vi "Motors.vi"(5 "Motors Active":refnum<vi>, 6 "Cluster":T1, 7 "Set":refnum<vi>, 8 "Error":refnum<vi>, 9 "Scan in Progress":refnum<vi>, 10 "EMERGENCY":refnum<vi>, 11 "QUIT":refnum<vi>) -> ()   [LabVIEW 2018]
uses:
  <vilib>/Utility/error.llb/DialogType.ctl
panel:
  out "Theta (deg)":refnum<vi>
  out "Z (mm)":refnum<vi>
  out "Y (mm)":refnum<vi>
  out "X (mm)":refnum<vi>
  out "Set?":bool
  out "Theta Go?":bool
  out "Z Go?":bool
  out "Y Go?":bool
  out "X Go?":bool
  out "Theta Go To (mm)":refnum<vi>
  out "Z Go To (mm)":refnum<vi>
  out "Y Go To (mm)":refnum<vi>
  out "X Go To (mm)":refnum<vi>
  out "Theta Go":refnum<vi>
  out "Z Go":refnum<vi>
  out "Y Go":refnum<vi>
  out "X Go":refnum<vi>
  out "Loop i":i32
  in  "Motors":enum32{"Controls", "Advanced Settings"}(tab)
  in  "Theta Speed (deg/s)":dbl=1.0 min=0.0
  in  "Z Speed (mm/s)":dbl=1.0 min=0.0
  in  "Y Speed (mm/s)":dbl=1.0 min=0.0
  in  "X Speed (mm/s)":dbl=1.0 min=0.0
  out "Status Z":string
  out "Status Theta":string
  out "Status Y":string
  out "Status X":string
  out "Z-Axis (mm)":dbl
  out "Theta (deg)":dbl
  out "Y-Axis (mm)":dbl
  out "X-Axis (mm)":dbl
  in  "theta+":bool
  in  "theta-":bool
  in  "Theta Go To":dbl
  in  "Theta Go":bool
  in  "x+":bool
  in  "x-":bool
  in  "X Go To":dbl
  in  "X Go":bool
  in  "y+":bool
  in  "y-":bool
  in  "Y Go To":dbl
  in  "Y Go":bool
  in  "z+":bool
  in  "z-":bool
  in  "Z Go To":dbl
  in  "Z Go":bool
  in  "Defined Positions":i32(listbox)
  in  "Go To Saved Position":bool
  in  "Delta X (mm)":dbl=1.0
  in  "Jog-Mode":bool
  in  "Delta Y (mm)":dbl=1.0
  in  "Delta Z (mm)":dbl=1.0
  in  "Delta Theta (deg)":dbl=1.0
  in  "Save New Position":bool
  in  "New Position Name":string
  in  "Delete Position":bool
  in  "Stop X":bool
  in  "Stop Y":bool
  in  "Stop Z":bool
  in  "Stop Theta":bool
  in  "Enable Motors":bool
  out "Motors Online":bool
  out "Motors Status":string
  out "Update Params":bool caption="Updating Motor Parameters"
  out "X Moving":bool caption="X"
  out "Y Moving":bool caption="Y"
  out "Z Moving":bool caption="Z"
  out "Theta Moving":bool caption="Theta"
  in  "Saved Positions":path=path "C:/LabView VIs/IPES SubVIs/saved_positions.txt"
  in  "Saved Limits":path=path "C:/LabView VIs/IPES SubVIs/saved_limits.txt"
  out "Theta Multiplier":u32=100 caption="steps/deg"
  out "Z Multiplier":u32=200 caption="steps/mm"
  out "Y Multiplier":u32=2000 caption="steps/mm"
  out "X Multiplier":u32=2000 caption="steps/mm"
  in  "Set Multipliers":bool
  in  "User Theta Mult":u32=100 caption="Theta" min=1
  in  "User Z Mult":u32=200 caption="Z" min=1
  in  "User Y Mult":u32=2000 caption="Y" min=1
  in  "User X Mult":u32=2000 caption="X" min=1
  in  "Set Joger":bool
  in  "Fast":dbl=200.0
  in  "Jogger Axis":u16(ring) items=["X (mm/s)", "Y (mm/s)", "Z (mm/s)", "Theta (deg/s)"]
  in  "Normal":dbl=200.0
  out "Y Jogger Fast Speed":dbl caption="mm/s"
  out "Y Jogger Normal Speed":dbl caption="mm/s"
  in  "Manual IO":bool
  in  "Reset Motors":bool caption="Load Previously Saved Parameters"
  in  "Redefine Origin":bool caption="Redefine Origin as Current Location"
  in  "Save Params":bool caption="Save Current Motor Parameters"
  in  "Find Datums":bool caption="Find Datums Nearest Hard Limits"
  in  "Use Datums":bool caption="Use Datums Nearest Hard Limits to Reset Origin"
  out "Manual Com":bool caption="Manual Communication is Active\n(Close Window Before Ending Program)"
  out "X Jogger Normal Speed":dbl caption="mm/s"
  out "X Jogger Fast Speed":dbl caption="mm/s"
  out "Z Jogger Normal Speed":dbl caption="mm/s"
  out "Z Jogger Fast Speed":dbl caption="mm/s"
  out "Theta Jogger Normal Speed":dbl caption="deg/s"
  out "Theta Jogger Fast Speed":dbl caption="deg/s"
  in  "Motors Port":refnum<visa-resource-name>="COM10"
  in  "User X Slew Speed":dbl=3.0 caption="X" min=0.4
  in  "User Y Slew Speed":dbl=3.0 caption="Y" min=0.4
  in  "User Z Slew Speed":dbl=2.0 caption="Z" min=0.5
  in  "User Theta Slew Speed":dbl=7.0 caption="Theta" min=1.0
  in  "X Set Slew Speed":bool
  in  "Y Set Slew Speed":bool
  in  "Z Set Slew Speed":bool
  in  "Theta Set Slew Speed":bool
  out "X Slew Speed":dbl caption="mm/s" min=0.0
  out "Y Slew Speed":dbl caption="mm/s" min=0.0
  out "Z Slew Speed":dbl caption="mm/s" min=0.0
  out "Theta Slew Speed":dbl caption="deg/s" min=0.0
  in  "Backlash X":u32=200 caption="X"
  in  "Backlash Y":u32=200 caption="Y"
  in  "Backlash Z":u32=50 caption="Z"
  in  "Backlash Theta":u32=50 caption="Theta"
  in  "Set Backlash":bool
  in  "Steps to Deactivate Hard Limit After Finding Datums":dbl=2000.0
  out "Theta Action":string
  out "Z Action":string
  out "Y Action":string
  out "X Action":string
  # "Status"
  # "Move Distance \n(Step Mode)"
  # "Remote Jogger Speeds"
  # "Encoder Multipliers"
  # "Motor Backlash Steps"
  # "Motor Speeds"
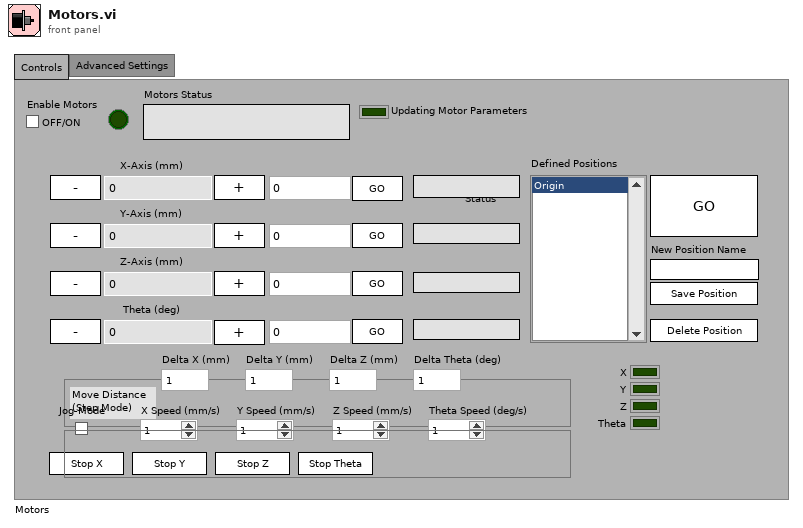
[diagram p1: front panel]
types:
  T1 = cluster{"X Go":refnum<vi>, "Y Go":refnum<vi>, "Z Go":refnum<vi>, "Theta Go":refnum<vi>, "X Go To (mm)":refnum<vi>, "Y Go To (mm)":refnum<vi>, "Z Go To (mm)":refnum<vi>, "Theta Go To (deg)":refnum<vi>, "X (mm)":refnum<vi>, "Y (mm)":refnum<vi>, "Z (mm)":refnum<vi>, "Theta (deg)":refnum<vi>}
  T2 = typedef "DialogType.ctl" = u16
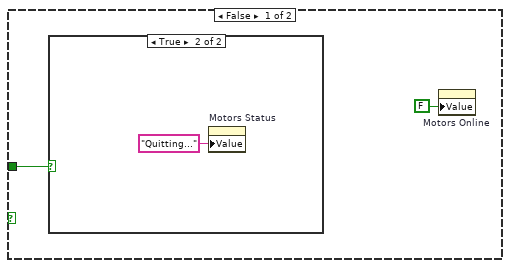
[diagram p2: hidden frame]
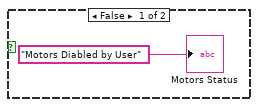
[diagram p3: hidden frame]
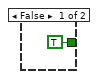
[diagram p10: hidden frame]
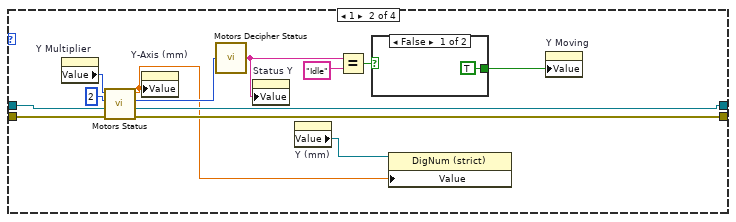
[diagram p11: hidden frame]
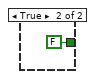
[diagram p12: hidden frame]
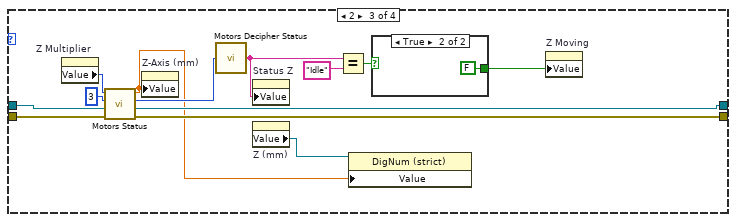
[diagram p13: hidden frame]
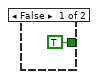
[diagram p14: hidden frame]
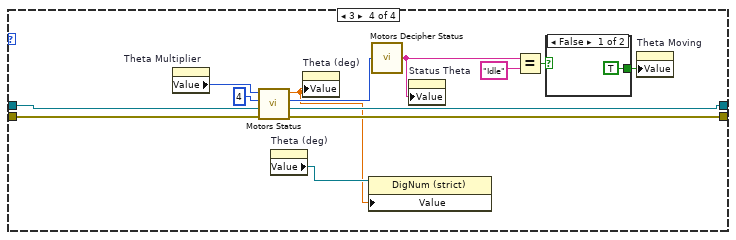
[diagram p15: hidden frame]
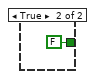
[diagram p16: hidden frame]
diagram:
  n1 = flat-sequence {
    frame #0 {
      w1 = FALSE ("Update Params")
      w2 = FALSE ("Visible")
      n2 = call "Motors Position Load.vi"() -> ("Positions"=w28:string[][])  [unwired: 2 in, 1 out]
      n3 = property on="Scan in Progress" class="LVObjRef (strict)"("Visible"=w2) -> ()  [unwired: 2 in, 2 out]
      n4 = property on="EMERGENCY" class="LVObjRef (strict)"("Visible"=w2) -> ()  [unwired: 2 in, 2 out]
      n5 = property on="Set" class="LVObjRef (strict)"("Visible"=w2) -> ()  [unwired: 2 in, 2 out]
      n6 = property on="Error" class="LVObjRef (strict)"("Visible"=w2) -> ()  [unwired: 2 in, 2 out]
      n7 = property on="Motors Active" class="LVObjRef (strict)"("Visible"=w2) -> ()  [unwired: 2 in, 2 out]
      n8 = property on="QUIT" class="LVObjRef (strict)"("Visible"=w2) -> ()  [unwired: 2 in, 2 out]
      n9 = property on="Loop i" class="DigNum (strict)"("Visible"=w2) -> ()  [unwired: 2 in, 2 out]
      n10 = property on="Set?" class="Bool (strict)"("Visible"=w2) -> ()  [unwired: 2 in, 2 out]
      n11 = property on="Z Go To (mm)" class="LVObjRef (strict)"("Visible"=w2) -> ()  [unwired: 2 in, 2 out]
      n12 = property on="Theta Go To (mm)" class="LVObjRef (strict)"("Visible"=w2) -> ()  [unwired: 2 in, 2 out]
      n13 = property on="Y Go To (mm)" class="LVObjRef (strict)"("Visible"=w2) -> ()  [unwired: 2 in, 2 out]
      n14 = property on="X Go To (mm)" class="LVObjRef (strict)"("Visible"=w2) -> ()  [unwired: 2 in, 2 out]
      n15 = property on="Y Go" class="LVObjRef (strict)"("Visible"=w2) -> ()  [unwired: 2 in, 2 out]
      n16 = property on="X Go" class="LVObjRef (strict)"("Visible"=w2) -> ()  [unwired: 2 in, 2 out]
      n17 = property on="Z Go" class="LVObjRef (strict)"("Visible"=w2) -> ()  [unwired: 2 in, 2 out]
      n18 = property on="Theta Go" class="LVObjRef (strict)"("Visible"=w2) -> ()  [unwired: 2 in, 2 out]
      n19 = property on="Cluster" class="Clust (strict)"("Visible"=w2) -> ()  [unwired: 2 in, 2 out]
      n20 = Array Subset(array=w28, index (row)=0 ("index"), length (row)=1 ("length"), index (col)=0 ("index")) -> (w24:string[][])  [unwired: 1 in]
      n21 = Unbundle("Cluster") -> ("X Go"=→"X Go":refnum<vi>, "Y Go"=→"Y Go":refnum<vi>, "Z Go"=→"Z Go":refnum<vi>, "Theta Go"=→"Theta Go":refnum<vi>, "X Go To (mm)"=→"X Go To (mm)":refnum<vi>, "Y Go To (mm)"=→"Y Go To (mm)":refnum<vi>, "Z Go To (mm)"=→"Z Go To (mm)":refnum<vi>, "Theta Go To (deg)"=→"Theta Go To (mm)":refnum<vi>, "X (mm)"=→"X (mm)":refnum<vi>, "Y (mm)"=→"Y (mm)":refnum<vi>, "Z (mm)"=→"Z (mm)":refnum<vi>, "Theta (deg)"=→"Theta (deg)":refnum<vi>)
      n22 = Initialize Array("", 1 ("dimension size")) -> (w21:string[])
      n23 = Index Array(array=w24) -> (element=w20:string[])  [unwired: 2 in]
      n24 = property on="X (mm)" class="LVObjRef (strict)"("Visible"=w2) -> ()  [unwired: 2 in, 2 out]
      n25 = property on="Z (mm)" class="LVObjRef (strict)"("Visible"=w2) -> ()  [unwired: 2 in, 2 out]
      n26 = property on="Y (mm)" class="LVObjRef (strict)"("Visible"=w2) -> ()  [unwired: 2 in, 2 out]
      n27 = property on="Theta (deg)" class="LVObjRef (strict)"("Visible"=w2) -> ()  [unwired: 2 in, 2 out]
      n28 = Insert Into Array(array=w21, new element=w20) -> (w19:string[])  [unwired: 1 in]
      n29 = property on="Enable Motors" class="Bool (strict)"("Value"=w1) -> ()  [unwired: 2 in, 2 out]
      n30 = property on="Update Params" class="Bool (strict)"("Value"=w1) -> ()  [unwired: 2 in, 2 out]
      n31 = property on="X Go?" class="Bool (strict)"("Visible"=w2) -> ()  [unwired: 2 in, 2 out]
      n32 = property on="Z Go?" class="Bool (strict)"("Visible"=w2) -> ()  [unwired: 2 in, 2 out]
      n33 = property on="Theta Go?" class="Bool (strict)"("Visible"=w2) -> ()  [unwired: 2 in, 2 out]
      n34 = property on="Y Go?" class="Bool (strict)"("Visible"=w2) -> ()  [unwired: 2 in, 2 out]
      n35 = Delete From Array(array=w19, index=0) -> (array with subset deleted=w17:string[])  [unwired: 1 in, 1 out]
      n36 = property on="Defined Positions" class="LstBox (strict)"("Item Names"=w17) -> ()  [unwired: 2 in, 2 out]
      n37 = property on="X Moving" class="Bool (strict)"("Value"=w1) -> ()  [unwired: 2 in, 2 out]
      n38 = property on="Y Moving" class="Bool (strict)"("Value"=w1) -> ()  [unwired: 2 in, 2 out]
      n39 = property on="Theta Moving" class="Bool (strict)"("Value"=w1) -> ()  [unwired: 2 in, 2 out]
      n40 = property on="Z Moving" class="Bool (strict)"("Value"=w1) -> ()  [unwired: 2 in, 2 out]
      "Motors Online" <- FALSE ("Motors Online")
      "Set?" <- FALSE ("Set?")
    }
    frame #1 {
      n41 = while {
        stop <- w36 stop-if-true
        n42 = property on="QUIT" class="LVObjRef (strict)"() -> ("Value"=w32:refnum<vi>)  [unwired: 2 in, 2 out]
        n43 = property class="Bool (strict)"(reference=w32) -> ("Value"=w34:bool)  [unwired: 1 in, 2 out]
        n44 = property class="Bool (strict)"(reference="QUIT") -> ("Value"=w36:bool)  [unwired: 1 in, 2 out]
        n45 = Not(x=w34) -> (.not. x?=w33:bool)
        n46 = And(x=w33, y="Enable Motors") -> (x .and. y?=w31:bool)
        n47 = case shown="True" w31 {
          tunnel: "Enable Motors" -> [w38 _]
          frame False {
            n48 = case shown="True" w38 {
              frame False {
                "Motors Status" <- "Motors Diabled by User" ("Motors Status")
              }
              frame True {
                n49 = property on="Motors Status" class="Str"("Value"="Quitting..." ("Motors Status")) -> ()  [unwired: 2 in, 2 out]
              }
            }
            n50 = property on="Motors Online" class="Bool (strict)"("Value"=FALSE ("Motors Online")) -> ()  [unwired: 2 in, 2 out]
          }
          frame True {
            n51 = call "Motors Open.vi"("VISA in"="Motors Port") -> ("error out"=w43:errorcluster, "VISA out"=w42:refnum<visa-resource-name>)  [unwired: 1 in]
            n52 = case shown="Error" w43 {
              selector: w43 -> [_ w1402]
              tunnel: w42 -> [w51 _]
              frame No Error {
                n53 = while {
                  tunnel: w51 -> [w57]
                  tunnel: [w55] -> w47
                  i -> [w56]
                  stop <- w65 stop-if-true
                  n54 = property on="Enable Motors" class="Bool (strict)"() -> ("Value"=w67:bool)  [unwired: 2 in, 2 out]
                  n55 = property on="QUIT" class="LVObjRef (strict)"() -> ("Value"=w64:refnum<vi>)  [unwired: 2 in, 2 out]
                  n56 = Not(x=w67) -> (.not. x?=w66:bool)
                  n57 = property class="Bool (strict)"(reference=w64) -> ("Value"=w63:bool)  [unwired: 1 in, 2 out]
                  n58 = property class="Bool (strict)"(reference="Scan in Progress") -> ("Value"=w61:bool)  [unwired: 1 in, 2 out]
                  n59 = property class="Bool (strict)"(reference="Set") -> ("Value"=w54:bool)  [unwired: 1 in, 2 out]
                  n60 = Or(x=w66, y=w63) -> (x .or. y?=w65:bool)
                  n61 = Not(x=w61) -> (.not. x?=w59:bool)
                  n62 = Or(x=w59, y=w54) -> (x .or. y?=w58:bool)
                  n63 = case shown="True" w58 {
                    tunnel: w57 -> [w68 w91]
                    tunnel: w56 -> [_ w182]
                    tunnel: [w68 w72] -> w55
                    tunnel: w54 -> [_ w93]
                    frame False {
                    }
                    frame True {
                      # "This loop checks every button consecutively (no particular order) to see if it has been pushed, and then executes the respective motor operation(s).  If a scan is running, the buttons are ignored and no operations are executed.  If the scan has called a <Set> operation, then the indicated motors are set to their indicated positions."
                      n64 = case shown="False" w93 {
                        tunnel: [w430 w436] -> w92
                        tunnel: w91 -> [w430 w436]
                        frame False {
                          # "A scan is not running.  If the user pushes a <# Go> button, then the # motor will move to the user-input position."
                          n65 = case shown="True" "Theta Go" {
                            selector: "Theta Go" -> [_ w432]
                            frame False {
                            }
                            frame True {
                              n66 = property on="Theta Go?" class="Bool (strict)"("Value"=w432) -> ()  [unwired: 2 in, 2 out]
                            }
                          }
                          n67 = case shown="True" "X Go" {
                            selector: "X Go" -> [_ w434]
                            frame False {
                            }
                            frame True {
                              n68 = property on="X Go?" class="Bool (strict)"("Value"=w434) -> ()  [unwired: 2 in, 2 out]
                            }
                          }
                          n69 = case shown="True" "Z Go" {
                            selector: "Z Go" -> [_ w431]
                            frame False {
                            }
                            frame True {
                              n70 = property on="Z Go?" class="Bool (strict)"("Value"=w431) -> ()  [unwired: 2 in, 2 out]
                            }
                          }
                          n71 = case shown="True" "Y Go" {
                            selector: "Y Go" -> [_ w433]
                            frame False {
                            }
                            frame True {
                              n72 = property on="Y Go?" class="Bool (strict)"("Value"=w433) -> ()  [unwired: 2 in, 2 out]
                            }
                          }
                        }
                        frame True {
                          # "<Set?> is a local variable that indicates that the global variable <Set> was True when the motor loop started.  We use it instead of just reading <Set> so as to avoid errors that may happen if another VI changes the state of <Set> part way through the motor loop being executed.  <Set?> will be set to True only if <Set> is True and <Set?> is False, thus the motor loop will execute exactly once."
                          n73 = property on="Set?" class="Bool (strict)"() -> ("Value"=w435:bool)  [unwired: 2 in, 2 out]
                          n74 = case shown="False" w435 {
                            frame False {
                              # "The global variables <# Go> are boolean flags that indacte if the position of the # motor should be set during a <Set> operation.  The global variables <# Go To> indicate the value of said position.  Both are copied to local variables to avoid errors if the the global variables are changed during the motor loop."
                              n75 = property on="Theta Go" class="LVObjRef (strict)"() -> ("Value"=w453:refnum<vi>)  [unwired: 2 in, 2 out]
                              n76 = property on="X Go" class="LVObjRef (strict)"() -> ("Value"=w447:refnum<vi>)  [unwired: 2 in, 2 out]
                              n77 = property on="Z Go" class="LVObjRef (strict)"() -> ("Value"=w451:refnum<vi>)  [unwired: 2 in, 2 out]
                              n78 = property on="Y Go" class="LVObjRef (strict)"() -> ("Value"=w445:refnum<vi>)  [unwired: 2 in, 2 out]
                              n79 = property on="Set?" class="Bool (strict)"("Value"=TRUE ("Set?")) -> ()  [unwired: 2 in, 2 out]
                              n80 = property class="Bool (strict)"(reference=w447) -> ("Value"=→"X Go?":bool)  [unwired: 1 in, 2 out]
                              n81 = property class="Bool (strict)"(reference=w451) -> ("Value"=→"Z Go?":bool)  [unwired: 1 in, 2 out]
                              n82 = property class="Bool (strict)"(reference=w445) -> ("Value"=→"Y Go?":bool)  [unwired: 1 in, 2 out]
                              n83 = property class="Bool (strict)"(reference=w453) -> ("Value"=→"Theta Go?":bool)  [unwired: 1 in, 2 out]
                              n84 = property on="Theta Go To (mm)" class="LVObjRef (strict)"() -> ("Value"=w448:refnum<vi>)  [unwired: 2 in, 2 out]
                              n85 = property on="Z Go To (mm)" class="LVObjRef (strict)"() -> ("Value"=w441:refnum<vi>)  [unwired: 2 in, 2 out]
                              n86 = property on="Y Go To (mm)" class="LVObjRef (strict)"() -> ("Value"=w440:refnum<vi>)  [unwired: 2 in, 2 out]
                              n87 = property on="X Go To (mm)" class="LVObjRef (strict)"() -> ("Value"=w438:refnum<vi>)  [unwired: 2 in, 2 out]
                              n88 = property class="DigNum (strict)"(reference=w441) -> ("Value"=w443:dbl)  [unwired: 1 in, 2 out]
                              n89 = property class="DigNum (strict)"(reference=w448) -> ("Value"=w449:dbl)  [unwired: 1 in, 2 out]
                              n90 = property class="DigNum (strict)"(reference=w440) -> ("Value"=w442:dbl)  [unwired: 1 in, 2 out]
                              n91 = property class="DigNum (strict)"(reference=w438) -> ("Value"=w439:dbl)  [unwired: 1 in, 2 out]
                              n92 = property on="Z Go To" class="DigNum (strict)"("Value"=w443) -> ()  [unwired: 2 in, 2 out]
                              n93 = property on="Theta Go To" class="DigNum (strict)"("Value"=w449) -> ()  [unwired: 2 in, 2 out]
                              n94 = property on="Y Go To" class="DigNum (strict)"("Value"=w442) -> ()  [unwired: 2 in, 2 out]
                              n95 = property on="X Go To" class="DigNum (strict)"("Value"=w439) -> ()  [unwired: 2 in, 2 out]
                            }
                            frame True {
                            }
                          }
                        }
                      }
                      n96 = property on="Error" class="LVObjRef (strict)"() -> ("Value"=w174:refnum<vi>)  [unwired: 2 in, 2 out]
                      n97 = property class="Clust (strict)"(reference=w174) -> ("Value"=w84:errorcluster)  [unwired: 1 in, 2 out]
                      n98 = property on="X Moving" class="Bool (strict)"() -> ("Value"=w98:bool)  [unwired: 2 in, 2 out]
                      n99 = property on="Y Moving" class="Bool (strict)"() -> ("Value"=w97:bool)  [unwired: 2 in, 2 out]
                      n100 = property on="Z Moving" class="Bool (strict)"() -> ("Value"=w96:bool)  [unwired: 2 in, 2 out]
                      n101 = property on="Theta Moving" class="Bool (strict)"() -> ("Value"=w95:bool)  [unwired: 2 in, 2 out]
                      n102 = Compound Arithmetic op=OR(w98, w97, w96, w95) -> (w94:bool)
                      n103 = case shown="False" "Save New Position" {
                        tunnel: w84 -> [w478 w497]
                        tunnel: [w478 w496] -> w103
                        frame False {
                        }
                        frame True {
                          # "Write the current position to file and make visible in the list of positions."
                          n104 = property on="Theta (deg)" class="DigNum (strict)"() -> ("Value"=w480:dbl)  [unwired: 2 in, 2 out]
                          n105 = property on="Saved Positions" class="Path"() -> ("Value"=w499:path)  [unwired: 2 in, 2 out]
                          n106 = property on="X-Axis (mm)" class="DigNum (strict)"() -> ("Value"=w483:dbl)  [unwired: 2 in, 2 out]
                          n107 = property on="Y-Axis (mm)" class="DigNum (strict)"() -> ("Value"=w482:dbl)  [unwired: 2 in, 2 out]
                          n108 = property on="Z-Axis (mm)" class="DigNum (strict)"() -> ("Value"=w481:dbl)  [unwired: 2 in, 2 out]
                          n109 = call "Motors Position Save.vi"("file path"=w499, "error in"=w497, "Position Name"="New Position Name", "Theta (deg)"=w480, "Z (mm)"=w481, "Y (mm)"=w482, "X (mm)"=w483) -> ("error out"=w498:errorcluster)  [unwired: 3 in]
                          n110 = call "Motors Position Load.vi"("error in"=w498, "file path"=w499) -> ("error out"=w496:errorcluster, "Positions"=w484:string[][])
                          n111 = Array Subset(array=w484, index (row)=0 ("index"), length (row)=1 ("length"), index (col)=0 ("index")) -> (w489:string[][])  [unwired: 1 in]
                          n112 = Initialize Array("", 1 ("dimension size")) -> (w490:string[])
                          n113 = Index Array(array=w489) -> (element=w492:string[])  [unwired: 2 in]
                          n114 = Insert Into Array(array=w490, new element=w492) -> (w493:string[])  [unwired: 1 in]
                          n115 = Delete From Array(array=w493, index=0) -> (array with subset deleted=w479:string[])  [unwired: 1 in, 1 out]
                          n116 = property on="Defined Positions" class="LstBox (strict)"("Item Names"=w479) -> ()  [unwired: 2 in, 2 out]
                        }
                      }
                      n117 = property class="Bool (strict)"(reference="Motors Active", "Value"=w94) -> ()  [unwired: 1 in, 2 out]
                      n118 = case shown="False" "Set Multipliers" {
                        frame False {
                        }
                        frame True {
                          # "Multipliers are the ratio of steps to mm (or deg) for each motor.  These are stored as local variables and used only by the GUI, i.e. not by the motor controllers."
                          "X Multiplier" <- "User X Mult"
                          "Y Multiplier" <- "User Y Mult"
                          "Z Multiplier" <- "User Z Mult"
                          "Theta Multiplier" <- "User Theta Mult"
                        }
                      }
                      n119 = case shown="False" "Delete Position" {
                        tunnel: w103 -> [w458 w476]
                        tunnel: [w458 w475] -> w102
                        frame False {
                        }
                        frame True {
                          # "Remove the selected position from the file and the list."
                          n120 = property on="Saved Positions" class="Path"() -> ("Value"=w461:path)  [unwired: 2 in, 2 out]
                          n121 = property on="Defined Positions" class="LstBox (strict)"() -> ("Value"=w460:i32)  [unwired: 2 in, 2 out]
                          n122 = call "Motors Position Load.vi"("error in"=w476, "file path"=w461) -> ("error out"=w477:errorcluster, "Positions"=w474:string[][])
                          n123 = Delete From Array(array=w474, index (col)=w460) -> (array with subset deleted=w473:string[][])  [unwired: 2 in, 1 out]
                          n124 = call "Motors Position Load.vi"("error in"=w477, "file path"=w461) -> ("error out"=w475:errorcluster, "Positions"=w462:string[][])
                          n125 = call "Motors Position Rewrite.vi"("file path"=w461, "Array of Positions"=w473) -> ()  [unwired: 9 in]
                          n126 = Array Subset(array=w462, index (row)=0 ("index"), length (row)=1 ("length"), index (col)=0 ("index")) -> (w467:string[][])  [unwired: 1 in]
                          n127 = Initialize Array("", 1 ("dimension size")) -> (w468:string[])
                          n128 = Index Array(array=w467) -> (element=w470:string[])  [unwired: 2 in]
                          n129 = Insert Into Array(array=w468, new element=w470) -> (w471:string[])  [unwired: 1 in]
                          n130 = Delete From Array(array=w471, index=0) -> (array with subset deleted=w459:string[])  [unwired: 1 in, 1 out]
                          n131 = property on="Defined Positions" class="LstBox (strict)"("Item Names"=w459) -> ()  [unwired: 2 in, 2 out]
                        }
                      }
                      n132 = case shown="False" "Stop X" {
                        tunnel: w102 -> [w1388 w1394]
                        tunnel: w92 -> [w1389 w1393]
                        tunnel: [w1389 w1391] -> w176
                        tunnel: [w1388 w1390] -> w177
                        frame False {
                        }
                        frame True {
                          # "The X motor stops moving immediately."
                          n133 = call "Motors Stop.vi"("error in"=w1394, "Axis"=1, "VISA in"=w1393) -> ("error out"=w1390:errorcluster, "VISA out"=w1391:refnum<visa-resource-name>)
                        }
                      }
                      n134 = case shown="False" "Stop Y" {
                        tunnel: w177 -> [w1381 w1387]
                        tunnel: w176 -> [w1382 w1386]
                        tunnel: [w1382 w1384] -> w178
                        tunnel: [w1381 w1383] -> w179
                        frame False {
                        }
                        frame True {
                          n135 = call "Motors Stop.vi"("error in"=w1387, "Axis"=2, "VISA in"=w1386) -> ("error out"=w1383:errorcluster, "VISA out"=w1384:refnum<visa-resource-name>)
                        }
                      }
                      n136 = case shown="False" "Stop Z" {
                        tunnel: w179 -> [w1374 w1380]
                        tunnel: w178 -> [w1375 w1379]
                        tunnel: [w1375 w1377] -> w180
                        tunnel: [w1374 w1376] -> w181
                        frame False {
                        }
                        frame True {
                          n137 = call "Motors Stop.vi"("error in"=w1380, "Axis"=3, "VISA in"=w1379) -> ("error out"=w1376:errorcluster, "VISA out"=w1377:refnum<visa-resource-name>)
                        }
                      }
                      n138 = case shown="True" "Stop Theta" {
                        tunnel: w181 -> [w1367 w1373]
                        tunnel: w180 -> [w1368 w1372]
                        tunnel: [w1368 w1370] -> w170
                        tunnel: [w1367 w1369] -> w169
                        frame False {
                        }
                        frame True {
                          n139 = call "Motors Stop.vi"("error in"=w1373, "Axis"=4, "VISA in"=w1372) -> ("error out"=w1369:errorcluster, "VISA out"=w1370:refnum<visa-resource-name>)
                        }
                      }
                      n140 = case shown="False" "Set Backlash" {
                        tunnel: [w1358 w1366] -> w166
                        tunnel: w170 -> [w1358 w1365]
                        tunnel: w169 -> [w1357 w1364]
                        tunnel: [w1357 w1363] -> w167
                        frame False {
                        }
                        frame True {
                          # "Set the number of steps to use for backlash correction."
                          n141 = call "Motors Backlash.vi"("X"="Backlash X", "Y"="Backlash Y", "VISA in"=w1365, "error in"=w1364, "Z"="Backlash Z", "Theta"="Backlash Theta") -> ("VISA out"=w1366:refnum<visa-resource-name>, "error out"=w1363:errorcluster)  [unwired: 2 in]
                        }
                      }
                      n142 = Or(x="x+", y="x-") -> (x .or. y?=w138:bool)
                      n143 = case shown="True" "Manual IO" {
                        tunnel: [w1340 w1347] -> w161
                        tunnel: [w1341 w1342] -> w162
                        tunnel: w166 -> [w1341 w1344]
                        tunnel: w167 -> [w1340 w1343]
                        frame False {
                        }
                        frame True {
                          # "Light the LED indicator and execute the Manual I/O subVI.  The VI quits if the user closes it or an <EMERGENCY> has occurred.  Turn the LED off when finished."
                          n144 = flat-sequence {
                            tunnel: [w1353] -> w1346
                            tunnel: [w1352] -> w1345
                            tunnel: w1344 -> [w1351]
                            tunnel: w1343 -> [w1350]
                            tunnel: [w1355] -> w1342
                            tunnel: [w1356] -> w1347
                            tunnel: w1346 -> [w1356]
                            tunnel: w1345 -> [w1355]
                            frame #0 {
                              "Manual Com" <- TRUE ("Manual Communication is Active\n(Close Before Ending Program) 2")
                            }
                            frame #1 {
                              n145 = call "Motors Manual IO.vi"("error in"=w1350, "Emergency Stop Reference"="EMERGENCY", "VISA in"=w1351) -> ("error out"=w1353:errorcluster, "VISA out"=w1352:refnum<visa-resource-name>)
                            }
                            frame #2 {
                              n146 = property on="Manual Com" class="Bool (strict)"("Value"=FALSE ("Manual Communication is Active\n(Close Before Ending Program)")) -> ()  [unwired: 2 in, 2 out]
                            }
                          }
                        }
                      }
                      n147 = property on="Update Params" class="Bool (strict)"() -> ("Value"=w105:bool)  [unwired: 2 in, 2 out]
                      n148 = case shown="False" "Reset Motors" {
                        tunnel: [w1334 w1339] -> w164
                        tunnel: [w1335 w1338] -> w163
                        tunnel: w162 -> [w1335 w1337]
                        tunnel: w161 -> [w1334 w1336]
                        frame False {
                        }
                        frame True {
                          # "Clears various abort conditions."
                          n149 = call "Motors Reset.vi"("error in"=w1336, "VISA in"=w1337) -> ("error out"=w1339:errorcluster, "VISA out"=w1338:refnum<visa-resource-name>)
                        }
                      }
                      n150 = Or(x="y+", y="y-") -> (x .or. y?=w135:bool)
                      n151 = case shown="3" "Jogger Axis" {
                        tunnel: [u32 1 u32 2 u32 3 u32 4] -> w157
                        tunnel: [w1303 w1309 w1315 w1321] -> w83
                        frame 0, Default {
                          w1299 = FALSE ("Visible")
                          w1300 = TRUE ("Visible")
                          w1301 = FALSE ("Visible")
                          w1302 = FALSE ("Visible")
                          # "Fancy GUI stuff."
                          n152 = property on="Z Jogger Fast Speed" class="DigNum (strict)"("Visible"=w1299) -> ()  [unwired: 2 in, 2 out]
                          n153 = property on="X Jogger Fast Speed" class="DigNum (strict)"("Visible"=w1300) -> ()  [unwired: 2 in, 2 out]
                          n154 = property on="Z Jogger Normal Speed" class="DigNum (strict)"("Visible"=w1299) -> ()  [unwired: 2 in, 2 out]
                          n155 = property on="Y Jogger Normal Speed" class="DigNum (strict)"("Visible"=w1302) -> ()  [unwired: 2 in, 2 out]
                          n156 = property on="Y Jogger Fast Speed" class="DigNum (strict)"("Visible"=w1302) -> ()  [unwired: 2 in, 2 out]
                          n157 = property on="X Jogger Normal Speed" class="DigNum (strict)"("Visible"=w1300) -> ()  [unwired: 2 in, 2 out]
                          n158 = property on="Theta Jogger Fast Speed" class="DigNum (strict)"("Visible"=w1301) -> ()  [unwired: 2 in, 2 out]
                          n159 = property on="Theta Jogger Normal Speed" class="DigNum (strict)"("Visible"=w1301) -> ()  [unwired: 2 in, 2 out]
                          n160 = property on="X Multiplier" class="DigNum (strict)"() -> ("Value"=w1303:u32)  [unwired: 2 in, 2 out]
                        }
                        frame 1 {
                          w1305 = FALSE ("Visible")
                          w1306 = FALSE ("Visible")
                          w1307 = FALSE ("Visible")
                          w1308 = TRUE ("Visible")
                          n161 = property on="Z Jogger Fast Speed" class="DigNum (strict)"("Visible"=w1305) -> ()  [unwired: 2 in, 2 out]
                          n162 = property on="X Jogger Fast Speed" class="DigNum (strict)"("Visible"=w1306) -> ()  [unwired: 2 in, 2 out]
                          n163 = property on="Z Jogger Normal Speed" class="DigNum (strict)"("Visible"=w1305) -> ()  [unwired: 2 in, 2 out]
                          n164 = property on="Y Jogger Normal Speed" class="DigNum (strict)"("Visible"=w1308) -> ()  [unwired: 2 in, 2 out]
                          n165 = property on="Y Jogger Fast Speed" class="DigNum (strict)"("Visible"=w1308) -> ()  [unwired: 2 in, 2 out]
                          n166 = property on="X Jogger Normal Speed" class="DigNum (strict)"("Visible"=w1306) -> ()  [unwired: 2 in, 2 out]
                          n167 = property on="Theta Jogger Fast Speed" class="DigNum (strict)"("Visible"=w1307) -> ()  [unwired: 2 in, 2 out]
                          n168 = property on="Theta Jogger Normal Speed" class="DigNum (strict)"("Visible"=w1307) -> ()  [unwired: 2 in, 2 out]
                          n169 = property on="Y Multiplier" class="DigNum (strict)"() -> ("Value"=w1309:u32)  [unwired: 2 in, 2 out]
                        }
                        frame 2 {
                          w1311 = TRUE ("Visible")
                          w1312 = FALSE ("Visible")
                          w1313 = FALSE ("Visible")
                          w1314 = FALSE ("Visible")
                          n170 = property on="Z Jogger Fast Speed" class="DigNum (strict)"("Visible"=w1311) -> ()  [unwired: 2 in, 2 out]
                          n171 = property on="X Jogger Fast Speed" class="DigNum (strict)"("Visible"=w1312) -> ()  [unwired: 2 in, 2 out]
                          n172 = property on="Z Jogger Normal Speed" class="DigNum (strict)"("Visible"=w1311) -> ()  [unwired: 2 in, 2 out]
                          n173 = property on="Y Jogger Normal Speed" class="DigNum (strict)"("Visible"=w1314) -> ()  [unwired: 2 in, 2 out]
                          n174 = property on="Y Jogger Fast Speed" class="DigNum (strict)"("Visible"=w1314) -> ()  [unwired: 2 in, 2 out]
                          n175 = property on="X Jogger Normal Speed" class="DigNum (strict)"("Visible"=w1312) -> ()  [unwired: 2 in, 2 out]
                          n176 = property on="Theta Jogger Fast Speed" class="DigNum (strict)"("Visible"=w1313) -> ()  [unwired: 2 in, 2 out]
                          n177 = property on="Theta Jogger Normal Speed" class="DigNum (strict)"("Visible"=w1313) -> ()  [unwired: 2 in, 2 out]
                          n178 = property on="Z Multiplier" class="DigNum (strict)"() -> ("Value"=w1315:u32)  [unwired: 2 in, 2 out]
                        }
                        frame 3 {
                          w1317 = FALSE ("Visible")
                          w1318 = FALSE ("Visible")
                          w1319 = TRUE ("Visible")
                          w1320 = FALSE ("Visible")
                          n179 = property on="Z Jogger Fast Speed" class="DigNum (strict)"("Visible"=w1317) -> ()  [unwired: 2 in, 2 out]
                          n180 = property on="X Jogger Fast Speed" class="DigNum (strict)"("Visible"=w1318) -> ()  [unwired: 2 in, 2 out]
                          n181 = property on="Z Jogger Normal Speed" class="DigNum (strict)"("Visible"=w1317) -> ()  [unwired: 2 in, 2 out]
                          n182 = property on="Y Jogger Normal Speed" class="DigNum (strict)"("Visible"=w1320) -> ()  [unwired: 2 in, 2 out]
                          n183 = property on="Y Jogger Fast Speed" class="DigNum (strict)"("Visible"=w1320) -> ()  [unwired: 2 in, 2 out]
                          n184 = property on="X Jogger Normal Speed" class="DigNum (strict)"("Visible"=w1318) -> ()  [unwired: 2 in, 2 out]
                          n185 = property on="Theta Jogger Fast Speed" class="DigNum (strict)"("Visible"=w1319) -> ()  [unwired: 2 in, 2 out]
                          n186 = property on="Theta Jogger Normal Speed" class="DigNum (strict)"("Visible"=w1319) -> ()  [unwired: 2 in, 2 out]
                          n187 = property on="Theta Multiplier" class="DigNum (strict)"() -> ("Value"=w1321:u32)  [unwired: 2 in, 2 out]
                        }
                      }
                      n188 = case shown="False" "Set Joger" {
                        tunnel: [w1324 w1333] -> w153
                        tunnel: [w1323 w1331] -> w154
                        tunnel: w83 -> [_ w1332]
                        tunnel: w164 -> [w1324 w1330]
                        tunnel: w163 -> [w1323 w1329]
                        tunnel: w157 -> [_ w1328]
                        frame False {
                        }
                        frame True {
                          # "Set Jogger speeds in steps/s."
                          n189 = property on="Update Params" class="Bool (strict)"("Value"=TRUE) -> ()  [unwired: 2 in, 2 out]
                          n190 = call "Motors Jogger Speed.vi"("Axis Multiplier"=w1332, "Axis"=w1328, "error in"=w1330, "VISA in"=w1329, "Fast Speed (mm or degree/sec)"="Fast", "Normal Speed (mm or degree/sec)"="Normal") -> ("error out"=w1333:errorcluster, "VISA out"=w1331:refnum<visa-resource-name>)  [unwired: 4 in]
                        }
                      }
                      n191 = case shown="False" "Redefine Origin" {
                        tunnel: [w1293 w1297] -> w156
                        tunnel: [w1294 w1298] -> w82
                        tunnel: w154 -> [w1294 w1296]
                        tunnel: w153 -> [w1293 w1295]
                        frame False {
                        }
                        frame True {
                          # "Sets current position to (0,0,0,0)."
                          n192 = call "Motors Redefine Origin.vi"("error in"=w1295, "VISA in"=w1296) -> ("error out"=w1297:errorcluster, "VISA out"=w1298:refnum<visa-resource-name>)
                        }
                      }
                      n193 = Or(x="z+", y="z-") -> (x .or. y?=w126:bool)
                      n194 = case shown="False" "Save Params" {
                        tunnel: w156 -> [w1288 w1292]
                        tunnel: [w1288 w1291] -> w151
                        tunnel: w82 -> [w1287 w1290]
                        tunnel: [w1287 w1289] -> w150
                        frame False {
                        }
                        frame True {
                          # "Tell the motor controllers to save all current parameters into their flash memory.  In case of an error or power failure, the motors' parameters will resume these values."
                          n195 = call "Motors Save.vi"("error in"=w1292, "VISA in"=w1290) -> ("error out"=w1291:errorcluster, "VISA out"=w1289:refnum<visa-resource-name>)
                        }
                      }
                      n196 = case shown="True" "Find Datums" {
                        tunnel: w151 -> [w1168 w1175]
                        tunnel: [w1168 w1173] -> w147
                        tunnel: [w1167 w1174] -> w148
                        tunnel: w150 -> [w1167 w1176]
                        frame False {
                        }
                        frame True {
                          n197 = flat-sequence {
                            tunnel: w1175 -> [w1179]
                            tunnel: w1176 -> [w1180]
                            tunnel: [w1180] -> w1172
                            tunnel: [w1179] -> w1171
                            tunnel: w1172 -> [w1209]
                            tunnel: w1171 -> [w1208]
                            tunnel: [w1204] -> w1170
                            tunnel: [w1203] -> w1169
                            tunnel: [w1285] -> w1173
                            tunnel: [w1286] -> w1174
                            tunnel: w1170 -> [w1286]
                            tunnel: w1169 -> [w1285]
                            frame #0 {
                              # "Deactivate the mouse and set status message."
                              n198 = call <vilib>:"Set Busy.vi"("disable click? (T)"=FALSE) -> ()  [unwired: 9 in, 2 out]
                              n199 = property on="Motors Status" class="Str"("Value"="Finding Datums Nearest Hard Limits\nThis May Take a Few Minutes" ("Status")) -> ()  [unwired: 2 in, 2 out]
                            }
                            frame #1 {
                              # "Start a subVI that moves each motor to the datum point nearest its hard limit.  Then update the motors' positions and status indicators.  Then save these positions."
                              n200 = property on="User X Slew Speed" class="DigNum (strict)"() -> ("Minimum"=w1191:dbl)  [unwired: 2 in, 2 out]
                              n201 = property on="User Y Slew Speed" class="DigNum (strict)"() -> ("Minimum"=w1188:dbl)  [unwired: 2 in, 2 out]
                              n202 = property on="X Multiplier" class="DigNum (strict)"() -> ("Value"=w1192:u32)  [unwired: 2 in, 2 out]
                              n203 = property on="Y Multiplier" class="DigNum (strict)"() -> ("Value"=w1189:u32)  [unwired: 2 in, 2 out]
                              n204 = property on="User Theta Slew Speed" class="DigNum (strict)"() -> ("Minimum"=w1183:dbl)  [unwired: 2 in, 2 out]
                              n205 = property on="User Z Slew Speed" class="DigNum (strict)"() -> ("Minimum"=w1186:dbl)  [unwired: 2 in, 2 out]
                              n206 = property on="Theta Multiplier" class="DigNum (strict)"() -> ("Value"=w1182:u32)  [unwired: 2 in, 2 out]
                              n207 = property on="Z Multiplier" class="DigNum (strict)"() -> ("Value"=w1185:u32)  [unwired: 2 in, 2 out]
                              n208 = Multiply(x=w1192, y=w1191) -> (x*y=w1190:dbl)
                              n209 = Multiply(x=w1189, y=w1188) -> (x*y=w1187:dbl)
                              n210 = Multiply(x=w1185, y=w1186) -> (x*y=w1184:dbl)
                              n211 = Multiply(x=w1182, y=w1183) -> (x*y=w1181:dbl)
                              n212 = call "Motors Find Datums.vi"("Creep Speed 4"=w1181, "Creep Speed 3"=w1184, "error in"=w1208, "Creep Speed 2"=w1187, "Creep Speed"=w1190, "VISA in"=w1209) -> ("error out"=w1205:errorcluster, "VISA out"=w1206:refnum<visa-resource-name>)
                              n213 = for {
                                N: 4 -> [_]
                                shift-right: [w1213] -> w1203
                                shift-left: w1205 -> [w1214]
                                tunnel: [w1211] -> w1195 mode=indexing
                                tunnel: w1206 -> [w1215]
                                tunnel: [w1212] -> w1204
                                i -> [w1210]
                                n214 = case shown="3" w1210 {
                                tunnel: w1214 -> [w1226 w1243 w1260 w1277]
                                tunnel: w1215 -> [w1227 w1244 w1261 w1278]
                                tunnel: [w1222 w1239 w1255 w1272] -> w1213
                                tunnel: [w1223 w1240 w1256 w1273] -> w1212
                                tunnel: [w1220 w1237 w1259 w1276] -> w1211
                                frame 0, Default {
                                w1221 = 1 ("Axis")
                                n215 = property on="X Multiplier" class="DigNum (strict)"() -> ("Value"=w1219:u32)  [unwired: 2 in, 2 out]
                                n216 = call "Motors Status.vi"("error in"=w1226, "VISA in"=w1227, "Axis"=w1221, "Axis Multiplier"=w1219) -> ("error out"=w1224:errorcluster, "VISA out"=w1225:refnum<visa-resource-name>, "OS"=w1230:i32, "Actual Position (mm or deg)"=→"X-Axis (mm)":dbl)  [unwired: 3 in]
                                n217 = call "Motors Decipher Status.vi"("OS"=w1230) -> ("Status"=w1217:string)
                                "Status X" <- w1217
                                n218 = Equal?(x=w1217, y="Idle") -> (x = y?=w1228:bool)
                                n219 = case shown="True" w1228 {
                                tunnel: [TRUE FALSE] -> w1216
                                frame False {
                                }
                                frame True {
                                }
                                }
                                "X Moving" <- w1216
                                n220 = call "Motors Datum Position.vi"("error in"=w1224, "VISA in"=w1225, "Axis"=w1221) -> ("error out"=w1222:errorcluster, "VISA out"=w1223:refnum<visa-resource-name>, "Datum Position (steps)"=w1220:string)  [unwired: 5 in]
                                }
                                frame 1 {
                                w1238 = 2 ("Axis")
                                n221 = property on="Y Multiplier" class="DigNum (strict)"() -> ("Value"=w1236:u32)  [unwired: 2 in, 2 out]
                                n222 = call "Motors Status.vi"("error in"=w1243, "VISA in"=w1244, "Axis"=w1238, "Axis Multiplier"=w1236) -> ("error out"=w1241:errorcluster, "VISA out"=w1242:refnum<visa-resource-name>, "OS"=w1247:i32, "Actual Position (mm or deg)"=→"Y-Axis (mm)":dbl)  [unwired: 3 in]
                                n223 = call "Motors Decipher Status.vi"("OS"=w1247) -> ("Status"=w1234:string)
                                "Status Y" <- w1234
                                n224 = Equal?(x=w1234, y="Idle") -> (x = y?=w1245:bool)
                                n225 = case shown="False" w1245 {
                                tunnel: [TRUE FALSE] -> w1233
                                frame False {
                                }
                                frame True {
                                }
                                }
                                "Y Moving" <- w1233
                                n226 = call "Motors Datum Position.vi"("error in"=w1241, "VISA in"=w1242, "Axis"=w1238) -> ("error out"=w1239:errorcluster, "VISA out"=w1240:refnum<visa-resource-name>, "Datum Position (steps)"=w1237:string)  [unwired: 5 in]
                                }
                                frame 2 {
                                w1254 = 3 ("Axis")
                                n227 = property on="Z Multiplier" class="DigNum (strict)"() -> ("Value"=w1253:u32)  [unwired: 2 in, 2 out]
                                n228 = call "Motors Status.vi"("error in"=w1260, "VISA in"=w1261, "Axis"=w1254, "Axis Multiplier"=w1253) -> ("error out"=w1257:errorcluster, "VISA out"=w1258:refnum<visa-resource-name>, "OS"=w1264:i32, "Actual Position (mm or deg)"=→"Z-Axis (mm)":dbl)  [unwired: 3 in]
                                n229 = call "Motors Decipher Status.vi"("OS"=w1264) -> ("Status"=w1251:string)
                                "Status Z" <- w1251
                                n230 = Equal?(x=w1251, y="Idle") -> (x = y?=w1262:bool)
                                n231 = case shown="False" w1262 {
                                tunnel: [TRUE FALSE] -> w1250
                                frame False {
                                }
                                frame True {
                                }
                                }
                                "Z Moving" <- w1250
                                n232 = call "Motors Datum Position.vi"("error in"=w1257, "VISA in"=w1258, "Axis"=w1254) -> ("error out"=w1255:errorcluster, "VISA out"=w1256:refnum<visa-resource-name>, "Datum Position (steps)"=w1259:string)  [unwired: 5 in]
                                }
                                frame 3 {
                                w1271 = 4 ("Axis")
                                n233 = property on="Theta Multiplier" class="DigNum (strict)"() -> ("Value"=w1270:u32)  [unwired: 2 in, 2 out]
                                n234 = call "Motors Status.vi"("error in"=w1277, "VISA in"=w1278, "Axis"=w1271, "Axis Multiplier"=w1270) -> ("error out"=w1274:errorcluster, "VISA out"=w1275:refnum<visa-resource-name>, "OS"=w1281:i32, "Actual Position (mm or deg)"=→"Theta (deg)":dbl)  [unwired: 3 in]
                                n235 = call "Motors Decipher Status.vi"("OS"=w1281) -> ("Status"=w1269:string)
                                "Status Theta" <- w1269
                                n236 = Equal?(x=w1269, y="Idle") -> (x = y?=w1279:bool)
                                n237 = case shown="True" w1279 {
                                tunnel: [TRUE FALSE] -> w1267
                                frame False {
                                }
                                frame True {
                                }
                                }
                                "Theta Moving" <- w1267
                                n238 = call "Motors Datum Position.vi"("error in"=w1274, "VISA in"=w1275, "Axis"=w1271) -> ("error out"=w1272:errorcluster, "VISA out"=w1273:refnum<visa-resource-name>, "Datum Position (steps)"=w1276:string)  [unwired: 5 in]
                                }
                                }
                              }
                              n239 = Build Array (concatenate)("Limits", w1195) -> (w1194:string[])
                              n240 = Initialize Array("", 0 ("dimension size"), 0 ("dimension size")) -> (w1201:string[][])
                              n241 = Build Array (concatenate)(w1194, w1201) -> (w1199:string[][])
                              n242 = Transpose 2D Array(2D array=w1199) -> (transposed array=w1198:string[][])
                              n243 = call "Motors Position Rewrite.vi"("file path"="Saved Limits", "Array of Positions"=w1198) -> ()  [unwired: 9 in]
                            }
                            frame #2 {
                              # "Reactivate mouse and resest status message."
                              n244 = call <vilib>:"Unset Busy.vi"() -> ()  [unwired: 11 in, 1 out]
                              n245 = property on="Motors Status" class="Str"("Value"="Running" ("Status")) -> ()  [unwired: 2 in, 2 out]
                            }
                          }
                        }
                      }
                      n246 = Or(x="theta+", y="theta-") -> (x .or. y?=w125:bool)
                      n247 = property on="Set?" class="Bool (strict)"() -> ("Value"=w85:bool)  [unwired: 2 in, 2 out]
                      n248 = case shown="False" "Use Datums" {
                        tunnel: [w964 w966] -> w139
                        tunnel: w147 -> [w964 w968]
                        tunnel: [w963 w965] -> w140
                        tunnel: w148 -> [w963 w969]
                        frame False {
                        }
                        frame True {
                          n249 = flat-sequence {
                            tunnel: w968 -> [w971]
                            tunnel: [w971] -> w967
                            tunnel: w969 -> [w993]
                            tunnel: w967 -> [w994]
                            tunnel: [w989] -> w966
                            tunnel: [w988] -> w965
                            frame #0 {
                              # "Deactivate mouse and set status message."
                              n250 = call <vilib>:"Set Busy.vi"() -> ()  [unwired: 10 in, 2 out]
                              n251 = property on="Motors Status" class="Str"("Value"="Finding Datums Nearest Hard Limits\nThis May Take a Few Minutes" ("Status")) -> ()  [unwired: 2 in, 2 out]
                            }
                            frame #1 {
                              # "Start a subVI that moves each motor to the datum point nearest its hard limit.  Then redefine the motors' current positions to the values stored in file.  Then update the motors' positions and status indicators."
                              n252 = property on="User X Slew Speed" class="DigNum (strict)"() -> ("Minimum"=w975:dbl)  [unwired: 2 in, 2 out]
                              n253 = property on="User Y Slew Speed" class="DigNum (strict)"() -> ("Minimum"=w974:dbl)  [unwired: 2 in, 2 out]
                              n254 = property on="X Multiplier" class="DigNum (strict)"() -> ("Value"=w983:u32)  [unwired: 2 in, 2 out]
                              n255 = property on="Y Multiplier" class="DigNum (strict)"() -> ("Value"=w982:u32)  [unwired: 2 in, 2 out]
                              n256 = property on="Saved Limits" class="Path"() -> ("Value"=w984:path)  [unwired: 2 in, 2 out]
                              n257 = property on="User Theta Slew Speed" class="DigNum (strict)"() -> ("Minimum"=w972:dbl)  [unwired: 2 in, 2 out]
                              n258 = property on="User Z Slew Speed" class="DigNum (strict)"() -> ("Minimum"=w973:dbl)  [unwired: 2 in, 2 out]
                              n259 = property on="Theta Multiplier" class="DigNum (strict)"() -> ("Value"=w980:u32)  [unwired: 2 in, 2 out]
                              n260 = property on="Z Multiplier" class="DigNum (strict)"() -> ("Value"=w981:u32)  [unwired: 2 in, 2 out]
                              n261 = Multiply(x=w983, y=w975) -> (x*y=w979:dbl)
                              n262 = Multiply(x=w982, y=w974) -> (x*y=w978:dbl)
                              n263 = Multiply(x=w981, y=w973) -> (x*y=w977:dbl)
                              n264 = Multiply(x=w980, y=w972) -> (x*y=w976:dbl)
                              n265 = call "Motors Find Datums.vi"("Creep Speed 4"=w976, "Creep Speed 3"=w977, "error in"=w994, "Creep Speed 2"=w978, "Creep Speed"=w979, "VISA in"=w993) -> ("error out"=w991:errorcluster, "VISA out"=w992:refnum<visa-resource-name>)
                              n266 = call "Motors Position Load.vi"("error in"=w991, "file path"=w984) -> ("error out"=w990:errorcluster, "Positions"=w987:string[][])
                              n267 = Delete From Array(array=w987, index (row)=0) -> (array with subset deleted=w985:string[][])  [unwired: 2 in, 1 out]
                              n268 = for {
                                shift-right: [w1005] -> w989
                                shift-left: w990 -> [w1006]
                                shift-right: [w1004] -> w988
                                shift-left: w992 -> [w1007]
                                tunnel: w985 -> [w1003] mode=indexing
                                tunnel: w975 -> [w998]
                                tunnel: w974 -> [w997]
                                tunnel: w973 -> [w996]
                                tunnel: w972 -> [w995]
                                i -> [w1000]
                                n269 = Index Array(array=w1003, index=0) -> (element=w1002:string)
                                n270 = Fract/Exp String To Number(string=w1002) -> (number=w1001:dbl)  [unwired: 3 in, 1 out]
                                n271 = case shown="0, Default" w1000 {
                                tunnel: w1006 -> [w1036 w1073 w1110 w1151]
                                tunnel: w1007 -> [w1037 w1074 w1111 w1152]
                                tunnel: [w1033 w1067 w1102 w1145] -> w1005
                                tunnel: [w1034 w1068 w1103 w1146] -> w1004
                                tunnel: w1001 -> [w1035 w1070 w1113 w1148]
                                tunnel: w998 -> [w1014 _ _ _]
                                tunnel: w997 -> [_ w1053 _ _]
                                tunnel: w996 -> [_ _ w1092 _]
                                tunnel: w995 -> [_ _ _ w1131]
                                frame 0, Default {
                                w1021 = u32 1 ("Axis Multiplier")
                                w1029 = 1 ("Axis")
                                n272 = property on="X Multiplier" class="DigNum (strict)"() -> ("Value"=w1016:u32)  [unwired: 2 in, 2 out]
                                n273 = call "Motors Status.vi"("error in"=w1036, "VISA in"=w1037, "Axis"=w1029, "Axis Multiplier"=w1016) -> ("error out"=w1025:errorcluster, "VISA out"=w1026:refnum<visa-resource-name>, "OS"=w1028:i32, "Actual Position (mm or deg)"=w1020:dbl)  [unwired: 3 in]
                                n274 = property on="X-Axis (mm)" class="DigNum (strict)"("Value"=w1020) -> ()  [unwired: 2 in, 2 out]
                                n275 = call "Motors Decipher Status.vi"("OS"=w1028) -> ("Status"=w1019:string)
                                n276 = call "Motors Position Redefine.vi"("Axis Multiplier"=w1021, "Axis"=w1029, "error in"=w1025, "VISA in"=w1026, "Position (mm or deg)"=w1035) -> ("error out"=w1024:errorcluster, "VISA out"=w1023:refnum<visa-resource-name>)  [unwired: 5 in]
                                n277 = property on="Status X" class="Str"("Value"=w1019) -> ()  [unwired: 2 in, 2 out]
                                n278 = property on="Steps to Deactivate Hard Limit After Finding Datums" class="DigNum (strict)"() -> ("Value"=w1017:dbl)  [unwired: 2 in, 2 out]
                                n279 = Equal?(x=w1019, y="Upper Hard Limit") -> (x = y?=w1018:bool)
                                n280 = Negate(x=w1017) -> (-x=w1022:dbl)
                                n281 = Divide(x=w1017, y=w1016) -> (x/y=w1015:dbl)
                                n282 = Divide(x=w1015, y=w1014) -> (x/y=w1009:dbl)
                                n283 = Multiply(x=w1009, y=1000.0) -> (x*y=w1010:dbl)
                                n284 = Round To Nearest(number=w1010) -> (nearest integer value=w1013:dbl)
                                n285 = Add(x=w1013, y=3000.0) -> (x+y=w1011:dbl)
                                n286 = case shown="True" w1018 {
                                tunnel: w1024 -> [w1039 w1047]
                                tunnel: [w1039 w1046] -> w1031
                                tunnel: w1023 -> [w1038 w1045]
                                tunnel: [w1038 w1044] -> w1030
                                tunnel: w1022 -> [_ w1043]
                                tunnel: w1029 -> [_ w1042]
                                tunnel: w1021 -> [_ w1041]
                                tunnel: w1011 -> [_ w1040]
                                frame False {
                                }
                                frame True {
                                n287 = call "Motors Move Relative.vi"("Axis Multiplier"=w1041, "Axis"=w1042, "error in"=w1047, "VISA in"=w1045, "Distance (mm)"=w1043) -> ("error out"=w1046:errorcluster, "VISA out"=w1044:refnum<visa-resource-name>)  [unwired: 5 in]
                                n288 = Wait (ms)(milliseconds to wait=w1040) -> ()  [unwired: 1 out]
                                }
                                }
                                n289 = call "Motors Move Absolute.vi"("Axis Multiplier"=w1016, "Axis"=w1029, "error in"=w1031, "VISA in"=w1030, "Position (mm or degree)"=0.0) -> ("error out"=w1033:errorcluster, "VISA out"=w1034:refnum<visa-resource-name>)  [unwired: 5 in]
                                }
                                frame 1 {
                                w1060 = u32 1 ("Axis Multiplier")
                                w1061 = 2 ("Axis")
                                n290 = property on="Y Multiplier" class="DigNum (strict)"() -> ("Value"=w1054:u32)  [unwired: 2 in, 2 out]
                                n291 = call "Motors Status.vi"("error in"=w1073, "VISA in"=w1074, "Axis"=w1061, "Axis Multiplier"=w1054) -> ("error out"=w1071:errorcluster, "VISA out"=w1072:refnum<visa-resource-name>, "OS"=w1077:i32, "Actual Position (mm or deg)"=w1059:dbl)  [unwired: 3 in]
                                n292 = property on="Y-Axis (mm)" class="DigNum (strict)"("Value"=w1059) -> ()  [unwired: 2 in, 2 out]
                                n293 = call "Motors Decipher Status.vi"("OS"=w1077) -> ("Status"=w1058:string)
                                n294 = call "Motors Position Redefine.vi"("Axis Multiplier"=w1060, "Axis"=w1061, "error in"=w1071, "VISA in"=w1072, "Position (mm or deg)"=w1070) -> ("error out"=w1064:errorcluster, "VISA out"=w1065:refnum<visa-resource-name>)  [unwired: 5 in]
                                n295 = property on="Status Y" class="Str"("Value"=w1058) -> ()  [unwired: 2 in, 2 out]
                                n296 = property on="Steps to Deactivate Hard Limit After Finding Datums" class="DigNum (strict)"() -> ("Value"=w1066:dbl)  [unwired: 2 in, 2 out]
                                n297 = Equal?(x=w1058, y="Upper Hard Limit") -> (x = y?=w1075:bool)
                                n298 = Negate(x=w1066) -> (-x=w1055:dbl)
                                n299 = Divide(x=w1055, y=w1054) -> (x/y=w1057:dbl)
                                n300 = Divide(x=w1057, y=w1053) -> (x/y=w1050:dbl)
                                n301 = Multiply(x=1000.0, y=w1050) -> (x*y=w1049:dbl)
                                n302 = Round To Nearest(number=w1049) -> (nearest integer value=w1056:dbl)
                                n303 = Add(x=w1056, y=3000.0) -> (x+y=w1052:dbl)
                                n304 = case shown="True" w1075 {
                                tunnel: w1065 -> [w1078 w1087]
                                tunnel: w1064 -> [w1079 w1086]
                                tunnel: [w1078 w1085] -> w1063
                                tunnel: [w1079 w1084] -> w1062
                                tunnel: w1055 -> [_ w1083]
                                tunnel: w1061 -> [_ w1082]
                                tunnel: w1060 -> [_ w1081]
                                tunnel: w1052 -> [_ w1080]
                                frame False {
                                }
                                frame True {
                                n305 = call "Motors Move Relative.vi"("Axis Multiplier"=w1081, "Axis"=w1082, "error in"=w1086, "VISA in"=w1087, "Distance (mm)"=w1083) -> ("error out"=w1084:errorcluster, "VISA out"=w1085:refnum<visa-resource-name>)  [unwired: 5 in]
                                n306 = Wait (ms)(milliseconds to wait=w1080) -> ()  [unwired: 1 out]
                                }
                                }
                                n307 = call "Motors Move Absolute.vi"("Axis Multiplier"=w1054, "Axis"=w1061, "error in"=w1062, "VISA in"=w1063, "Position (mm or degree)"=0.0) -> ("error out"=w1067:errorcluster, "VISA out"=w1068:refnum<visa-resource-name>)  [unwired: 5 in]
                                }
                                frame 2 {
                                w1100 = u32 1 ("Axis Multiplier")
                                w1101 = 3 ("Axis")
                                n308 = property on="Z Multiplier" class="DigNum (strict)"() -> ("Value"=w1093:u32)  [unwired: 2 in, 2 out]
                                n309 = call "Motors Status.vi"("error in"=w1110, "VISA in"=w1111, "Axis"=w1101, "Axis Multiplier"=w1093) -> ("error out"=w1108:errorcluster, "VISA out"=w1109:refnum<visa-resource-name>, "OS"=w1116:i32, "Actual Position (mm or deg)"=w1099:dbl)  [unwired: 3 in]
                                n310 = property on="Z-Axis (mm)" class="DigNum (strict)"("Value"=w1099) -> ()  [unwired: 2 in, 2 out]
                                n311 = call "Motors Decipher Status.vi"("OS"=w1116) -> ("Status"=w1098:string)
                                n312 = call "Motors Position Redefine.vi"("Axis Multiplier"=w1100, "Axis"=w1101, "error in"=w1108, "VISA in"=w1109, "Position (mm or deg)"=w1113) -> ("error out"=w1106:errorcluster, "VISA out"=w1107:refnum<visa-resource-name>)  [unwired: 5 in]
                                n313 = property on="Status Z" class="Str"("Value"=w1098) -> ()  [unwired: 2 in, 2 out]
                                n314 = property on="Steps to Deactivate Hard Limit After Finding Datums" class="DigNum (strict)"() -> ("Value"=w1094:dbl)  [unwired: 2 in, 2 out]
                                n315 = Equal?(x=w1098, y="Upper Hard Limit") -> (x = y?=w1114:bool)
                                n316 = Divide(x=w1094, y=w1093) -> (x/y=w1097:dbl)
                                n317 = Divide(x=w1097, y=w1092) -> (x/y=w1089:dbl)
                                n318 = Multiply(x=1000.0, y=w1089) -> (x*y=w1090:dbl)
                                n319 = Round To Nearest(number=w1090) -> (nearest integer value=w1096:dbl)
                                n320 = Add(x=w1096, y=3000.0) -> (x+y=w1091:dbl)
                                n321 = case shown="True" w1114 {
                                tunnel: w1107 -> [w1117 w1126]
                                tunnel: w1106 -> [w1118 w1125]
                                tunnel: [w1117 w1124] -> w1105
                                tunnel: [w1118 w1123] -> w1104
                                tunnel: w1094 -> [_ w1122]
                                tunnel: w1101 -> [_ w1121]
                                tunnel: w1100 -> [_ w1120]
                                tunnel: w1091 -> [_ w1119]
                                frame False {
                                }
                                frame True {
                                n322 = call "Motors Move Relative.vi"("Axis Multiplier"=w1120, "Axis"=w1121, "error in"=w1125, "VISA in"=w1126, "Distance (mm)"=w1122) -> ("error out"=w1123:errorcluster, "VISA out"=w1124:refnum<visa-resource-name>)  [unwired: 5 in]
                                n323 = Wait (ms)(milliseconds to wait=w1119) -> ()  [unwired: 1 out]
                                }
                                }
                                n324 = call "Motors Move Absolute.vi"("Axis Multiplier"=w1093, "Axis"=w1101, "error in"=w1104, "VISA in"=w1105, "Position (mm or degree)"=0.0) -> ("error out"=w1102:errorcluster, "VISA out"=w1103:refnum<visa-resource-name>)  [unwired: 5 in]
                                }
                                frame 3 {
                                w1139 = u32 1 ("Axis Multiplier")
                                w1140 = 4 ("Axis")
                                n325 = property on="Theta Multiplier" class="DigNum (strict)"() -> ("Value"=w1132:u32)  [unwired: 2 in, 2 out]
                                n326 = call "Motors Status.vi"("error in"=w1151, "VISA in"=w1152, "Axis"=w1140, "Axis Multiplier"=w1132) -> ("error out"=w1149:errorcluster, "VISA out"=w1150:refnum<visa-resource-name>, "OS"=w1155:i32, "Actual Position (mm or deg)"=w1138:dbl)  [unwired: 3 in]
                                n327 = property on="Theta (deg)" class="DigNum (strict)"("Value"=w1138) -> ()  [unwired: 2 in, 2 out]
                                n328 = call "Motors Position Redefine.vi"("Axis Multiplier"=w1139, "Axis"=w1140, "error in"=w1149, "VISA in"=w1150, "Position (mm or deg)"=w1148) -> ("error out"=w1143:errorcluster, "VISA out"=w1144:refnum<visa-resource-name>)  [unwired: 5 in]
                                n329 = call "Motors Decipher Status.vi"("OS"=w1155) -> ("Status"=w1137:string)
                                n330 = property on="Status Theta" class="Str"("Value"=w1137) -> ()  [unwired: 2 in, 2 out]
                                n331 = Equal?(x=w1137, y="Upper Hard Limit") -> (x = y?=w1153:bool)
                                n332 = Divide(x="Steps to Deactivate Hard Limit After Finding Datums", y=w1132) -> (x/y=w1136:dbl)
                                n333 = Divide(x=w1136, y=w1131) -> (x/y=w1128:dbl)
                                n334 = Multiply(x=1000.0, y=w1128) -> (x*y=w1129:dbl)
                                n335 = Round To Nearest(number=w1129) -> (nearest integer value=w1135:dbl)
                                n336 = Add(x=w1135, y=3000.0) -> (x+y=w1130:dbl)
                                n337 = case shown="True" w1153 {
                                tunnel: w1144 -> [w1157 w1165]
                                tunnel: w1143 -> [w1156 w1164]
                                tunnel: [w1157 w1163] -> w1142
                                tunnel: [w1156 w1162] -> w1141
                                tunnel: "Steps to Deactivate Hard Limit After Finding Datums" -> [_ w1161]
                                tunnel: w1140 -> [_ w1160]
                                tunnel: w1139 -> [_ w1159]
                                tunnel: w1130 -> [_ w1158]
                                frame False {
                                }
                                frame True {
                                n338 = call "Motors Move Relative.vi"("Axis Multiplier"=w1159, "Axis"=w1160, "error in"=w1164, "VISA in"=w1165, "Distance (mm)"=w1161) -> ("error out"=w1162:errorcluster, "VISA out"=w1163:refnum<visa-resource-name>)  [unwired: 5 in]
                                n339 = Wait (ms)(milliseconds to wait=w1158) -> ()  [unwired: 1 out]
                                }
                                }
                                n340 = call "Motors Move Absolute.vi"("Axis Multiplier"=w1132, "Axis"=w1140, "error in"=w1141, "VISA in"=w1142, "Position (mm or degree)"=0.0) -> ("error out"=w1145:errorcluster, "VISA out"=w1146:refnum<visa-resource-name>)  [unwired: 5 in]
                                }
                                }
                              }
                            }
                            frame #2 {
                              # "Reactivate the mouse and reset the status message."
                              n341 = call <vilib>:"Unset Busy.vi"() -> ()  [unwired: 11 in, 1 out]
                              n342 = property on="Motors Status" class="Str"("Value"="Running" ("Status")) -> ()  [unwired: 2 in, 2 out]
                            }
                          }
                        }
                      }
                      n343 = Quotient & Remainder(x=w182, y=4) -> (x-y*floor(x/y)=w86:i32)  [unwired: 1 out]
                      n344 = property on="X Go?" class="Bool (strict)"() -> ("Value"=w90:bool)  [unwired: 2 in, 2 out]
                      n345 = property on="Set?" class="Bool (strict)"() -> ("Value"=w69:bool)  [unwired: 2 in, 2 out]
                      n346 = case shown="True" w90 {
                        tunnel: w140 -> [w952 w958]
                        tunnel: w139 -> [w951 w961]
                        tunnel: [w952 w959] -> w141
                        tunnel: [w951 w960] -> w81
                        tunnel: w69 -> [_ w953]
                        frame False {
                        }
                        frame True {
                          # "This case is activated if (there is a scan running AND <Set> is True AND <X Go> is True) OR (there is not a scan running AND the user pushed the <X Go> button)."
                          n347 = case shown="False" w953 {
                            frame False {
                              n348 = property on="X Go?" class="Bool (strict)"("Value"=FALSE ("X Go?")) -> ()  [unwired: 2 in, 2 out]
                            }
                            frame True {
                            }
                          }
                          n349 = property on="X Multiplier" class="DigNum (strict)"() -> ("Value"=w956:u32)  [unwired: 2 in, 2 out]
                          n350 = property on="X Moving" class="Bool (strict)"("Value"=TRUE ("X Moving")) -> ()  [unwired: 2 in, 2 out]
                          n351 = call "Motors Move Absolute.vi"("Axis Multiplier"=w956, "Axis"=u32 1, "error in"=w961, "VISA in"=w958, "Position (mm or degree)"="X Go To") -> ("error out"=w960:errorcluster, "VISA out"=w959:refnum<visa-resource-name>)  [unwired: 5 in]
                        }
                      }
                      n352 = property on="Y Go?" class="Bool (strict)"() -> ("Value"=w89:bool)  [unwired: 2 in, 2 out]
                      n353 = case shown="False" w89 {
                        tunnel: w141 -> [w940 w946]
                        tunnel: w81 -> [w939 w949]
                        tunnel: [w940 w947] -> w142
                        tunnel: [w939 w948] -> w143
                        tunnel: w69 -> [_ w941]
                        frame False {
                        }
                        frame True {
                          # "<# Moving> must be set to True at this point.  If Motor # is already at <# Go To>, then the motor won't move, the status won't change from Idle, and the scan will wait around forever for something to happen."
                          n354 = case shown="False" w941 {
                            frame False {
                              n355 = property on="Y Go?" class="Bool (strict)"("Value"=FALSE ("Y Go?")) -> ()  [unwired: 2 in, 2 out]
                            }
                            frame True {
                            }
                          }
                          n356 = property on="Y Multiplier" class="DigNum (strict)"() -> ("Value"=w944:u32)  [unwired: 2 in, 2 out]
                          n357 = property on="Y Moving" class="Bool (strict)"("Value"=TRUE ("Y Moving")) -> ()  [unwired: 2 in, 2 out]
                          n358 = call "Motors Move Absolute.vi"("Axis Multiplier"=w944, "Axis"=u32 2, "error in"=w949, "VISA in"=w946, "Position (mm or degree)"="Y Go To") -> ("error out"=w948:errorcluster, "VISA out"=w947:refnum<visa-resource-name>)  [unwired: 5 in]
                        }
                      }
                      n359 = property on="Z Go?" class="Bool (strict)"() -> ("Value"=w80:bool)  [unwired: 2 in, 2 out]
                      n360 = case shown="False" w80 {
                        tunnel: w142 -> [w928 w933]
                        tunnel: w143 -> [w927 w937]
                        tunnel: [w928 w935] -> w144
                        tunnel: [w927 w936] -> w145
                        tunnel: w69 -> [_ w929]
                        frame False {
                        }
                        frame True {
                          n361 = case shown="False" w929 {
                            frame False {
                              n362 = property on="Z Go?" class="Bool (strict)"("Value"=FALSE ("Z Go?")) -> ()  [unwired: 2 in, 2 out]
                            }
                            frame True {
                            }
                          }
                          n363 = property on="Z Multiplier" class="DigNum (strict)"() -> ("Value"=w932:u32)  [unwired: 2 in, 2 out]
                          n364 = property on="Z Moving" class="Bool (strict)"("Value"=TRUE ("Z Moving")) -> ()  [unwired: 2 in, 2 out]
                          n365 = call "Motors Move Absolute.vi"("Axis Multiplier"=w932, "Axis"=u32 3, "error in"=w937, "VISA in"=w933, "Position (mm or degree)"="Z Go To") -> ("error out"=w936:errorcluster, "VISA out"=w935:refnum<visa-resource-name>)  [unwired: 5 in]
                        }
                      }
                      n366 = property on="Theta Go?" class="Bool (strict)"() -> ("Value"=w88:bool)  [unwired: 2 in, 2 out]
                      n367 = case shown="True" w88 {
                        tunnel: w144 -> [w915 w922]
                        tunnel: w145 -> [w916 w925]
                        tunnel: [w916 w924] -> w74
                        tunnel: [w915 w923] -> w75
                        tunnel: w69 -> [_ w917]
                        frame False {
                        }
                        frame True {
                          n368 = case shown="False" w917 {
                            frame False {
                              n369 = property on="Theta Go?" class="Bool (strict)"("Value"=FALSE ("Theta Go?")) -> ()  [unwired: 2 in, 2 out]
                            }
                            frame True {
                            }
                          }
                          n370 = property on="Theta Multiplier" class="DigNum (strict)"() -> ("Value"=w920:u32)  [unwired: 2 in, 2 out]
                          n371 = property on="Theta Moving" class="Bool (strict)"("Value"=TRUE ("Theta Moving")) -> ()  [unwired: 2 in, 2 out]
                          n372 = call "Motors Move Absolute.vi"("Axis Multiplier"=w920, "Axis"=u32 4, "error in"=w925, "VISA in"=w922, "Position (mm or degree)"="Theta Go To") -> ("error out"=w924:errorcluster, "VISA out"=w923:refnum<visa-resource-name>)  [unwired: 5 in]
                        }
                      }
                      n373 = case shown="False" w138 {
                        tunnel: w75 -> [w847 w853]
                        tunnel: w74 -> [w846 w852]
                        tunnel: [w847 w851] -> w134
                        tunnel: [w846 w850] -> w133
                        frame False {
                        }
                        frame True {
                          n374 = flat-sequence {
                            tunnel: w853 -> [w859]
                            tunnel: w852 -> [w858]
                            tunnel: [w857] -> w849
                            tunnel: [w856] -> w848
                            tunnel: [w913] -> w850
                            tunnel: [w914] -> w851
                            tunnel: w849 -> [w914]
                            tunnel: w848 -> [w913]
                            frame #0 {
                              n375 = property on="X Multiplier" class="DigNum (strict)"() -> ("Value"=w854:u32)  [unwired: 2 in, 2 out]
                              n376 = case shown="True" "Jog-Mode" {
                                tunnel: w859 -> [w865 w887]
                                tunnel: w858 -> [w862 w890]
                                tunnel: [w864 w892] -> w857
                                tunnel: [w863 w891] -> w856
                                tunnel: w854 -> [w860 w884]
                                frame False {
                                # "Only initiate a move if X starts stationary (to avoid erroneous perpetual motion)."
                                n377 = property on="X Moving" class="Bool (strict)"() -> ("Value"=w861:bool)  [unwired: 2 in, 2 out]
                                n378 = case shown="False" w861 {
                                tunnel: w865 -> [w871 w881]
                                tunnel: w862 -> [w875 w880]
                                tunnel: [w873 w881] -> w864
                                tunnel: [w874 w880] -> w863
                                tunnel: w860 -> [w868 _]
                                frame False {
                                # "Move by Delta X."
                                n379 = property on="x-" class="Bool (strict)"() -> ("Value"=w867:bool)  [unwired: 2 in, 2 out]
                                n380 = property on="X Moving" class="Bool (strict)"("Value"=TRUE ("X Moving")) -> ()  [unwired: 2 in, 2 out]
                                n381 = case shown="True" w867 {
                                tunnel: "Delta X (mm)" -> [w876 w878]
                                tunnel: [w876 w877] -> w872
                                frame False {
                                }
                                frame True {
                                n382 = Multiply(x=w878, y=-1.0) -> (x*y=w877:dbl)
                                }
                                }
                                n383 = call "Motors Move Relative.vi"("Axis Multiplier"=w868, "Axis"=1, "error in"=w875, "VISA in"=w871, "Distance (mm)"=w872) -> ("error out"=w874:errorcluster, "VISA out"=w873:refnum<visa-resource-name>)  [unwired: 5 in]
                                }
                                frame True {
                                }
                                }
                                }
                                frame True {
                                w885 = 1 ("Axis")
                                # "Move until the +/- button is released."
                                n384 = property on="x-" class="Bool (strict)"() -> ("Value"=w882:bool)  [unwired: 2 in, 2 out]
                                n385 = case shown="True" w882 {
                                tunnel: "X Speed (mm/s)" -> [w907 w909]
                                tunnel: [w907 w908] -> w888
                                frame False {
                                }
                                frame True {
                                n386 = Multiply(x=w909, y=-1.0) -> (x*y=w908:dbl)
                                }
                                }
                                n387 = call "Motors Move Constant Velocity.vi"("Axis Multiplier"=w884, "Axis"=w885, "error in"=w890, "VISA in"=w887, "Speed (mm/s)"=w888) -> ("error out"=w889:errorcluster, "VISA out"=w886:refnum<visa-resource-name>)  [unwired: 5 in]
                                n388 = while {
                                tunnel: w886 -> [w900]
                                tunnel: [w902] -> w894
                                tunnel: w889 -> [w903]
                                tunnel: [w901] -> w893
                                tunnel: w884 -> [w899]
                                stop <- w906 continue-if-true
                                n389 = property on="x+" class="Bool (strict)"() -> ("Value"=w898:bool)  [unwired: 2 in, 2 out]
                                n390 = property on="x-" class="Bool (strict)"() -> ("Value"=w897:bool)  [unwired: 2 in, 2 out]
                                n391 = Or(x=w898, y=w897) -> (x .or. y?=w906:bool)
                                n392 = call "Motors Status.vi"("error in"=w903, "VISA in"=w900, "Axis"=1, "Axis Multiplier"=w899) -> ("error out"=w901:errorcluster, "VISA out"=w902:refnum<visa-resource-name>, "OS"=w904:i32, "Actual Position (mm or deg)"=w895:dbl)  [unwired: 3 in]
                                n393 = property on="X-Axis (mm)" class="DigNum (strict)"("Value"=w895) -> ()  [unwired: 2 in, 2 out]
                                n394 = call "Motors Decipher Status.vi"("OS"=w904) -> ("Status"=w896:string)
                                n395 = property on="Status X" class="Str"("Value"=w896) -> ()  [unwired: 2 in, 2 out]
                                }
                                n396 = call "Motors Stop.vi"("error in"=w893, "Axis"=w885, "VISA in"=w894) -> ("error out"=w891:errorcluster, "VISA out"=w892:refnum<visa-resource-name>)
                                }
                              }
                            }
                            frame #1 {
                              n397 = property on="x+" class="Bool (strict)"("Value"=FALSE) -> ()  [unwired: 2 in, 2 out]
                              n398 = property on="x-" class="Bool (strict)"("Value"=FALSE) -> ()  [unwired: 2 in, 2 out]
                            }
                          }
                        }
                      }
                      n399 = case shown="False" w135 {
                        tunnel: w134 -> [w778 w784]
                        tunnel: w133 -> [w777 w783]
                        tunnel: [w778 w782] -> w130
                        tunnel: [w777 w781] -> w129
                        frame False {
                        }
                        frame True {
                          n400 = flat-sequence {
                            tunnel: w784 -> [w790]
                            tunnel: w783 -> [w789]
                            tunnel: [w788] -> w780
                            tunnel: [w787] -> w779
                            tunnel: [w844] -> w781
                            tunnel: [w845] -> w782
                            tunnel: w780 -> [w845]
                            tunnel: w779 -> [w844]
                            frame #0 {
                              n401 = property on="Y Multiplier" class="DigNum (strict)"() -> ("Value"=w785:u32)  [unwired: 2 in, 2 out]
                              n402 = property on="Jog-Mode" class="Bool (strict)"() -> ("Value"=w786:bool)  [unwired: 2 in, 2 out]
                              n403 = case shown="True" w786 {
                                tunnel: w790 -> [w796 w818]
                                tunnel: w789 -> [w795 w821]
                                tunnel: [w794 w823] -> w788
                                tunnel: [w793 w822] -> w787
                                tunnel: w785 -> [w792 w814]
                                frame False {
                                n404 = property on="Y Moving" class="Bool (strict)"() -> ("Value"=w791:bool)  [unwired: 2 in, 2 out]
                                n405 = case shown="False" w791 {
                                tunnel: w796 -> [w803 w812]
                                tunnel: w795 -> [w806 w811]
                                tunnel: [w804 w812] -> w794
                                tunnel: [w805 w811] -> w793
                                tunnel: w792 -> [w800 _]
                                frame False {
                                n406 = property on="Y Moving" class="Bool (strict)"("Value"=TRUE ("Y Moving")) -> ()  [unwired: 2 in, 2 out]
                                n407 = property on="y-" class="Bool (strict)"() -> ("Value"=w798:bool)  [unwired: 2 in, 2 out]
                                n408 = case shown="True" w798 {
                                tunnel: "Delta Y (mm)" -> [w807 w809]
                                tunnel: [w807 w808] -> w802
                                frame False {
                                }
                                frame True {
                                n409 = Multiply(x=w809, y=-1.0) -> (x*y=w808:dbl)
                                }
                                }
                                n410 = call "Motors Move Relative.vi"("Axis Multiplier"=w800, "Axis"=2, "error in"=w806, "VISA in"=w803, "Distance (mm)"=w802) -> ("error out"=w805:errorcluster, "VISA out"=w804:refnum<visa-resource-name>)  [unwired: 5 in]
                                }
                                frame True {
                                }
                                }
                                }
                                frame True {
                                w816 = 2 ("Axis")
                                n411 = property on="y-" class="Bool (strict)"() -> ("Value"=w815:bool)  [unwired: 2 in, 2 out]
                                n412 = case shown="True" w815 {
                                tunnel: "Y Speed (mm/s)" -> [w838 w840]
                                tunnel: [w838 w839] -> w819
                                frame False {
                                }
                                frame True {
                                n413 = Multiply(x=w840, y=-1.0) -> (x*y=w839:dbl)
                                }
                                }
                                n414 = call "Motors Move Constant Velocity.vi"("Axis Multiplier"=w814, "Axis"=w816, "error in"=w821, "VISA in"=w818, "Speed (mm/s)"=w819) -> ("error out"=w820:errorcluster, "VISA out"=w817:refnum<visa-resource-name>)  [unwired: 5 in]
                                n415 = while {
                                tunnel: w817 -> [w832]
                                tunnel: [w831] -> w825
                                tunnel: w820 -> [w834]
                                tunnel: [w833] -> w824
                                tunnel: w814 -> [w830]
                                stop <- w837 continue-if-true
                                n416 = property on="y+" class="Bool (strict)"() -> ("Value"=w829:bool)  [unwired: 2 in, 2 out]
                                n417 = property on="y-" class="Bool (strict)"() -> ("Value"=w828:bool)  [unwired: 2 in, 2 out]
                                n418 = Or(x=w829, y=w828) -> (x .or. y?=w837:bool)
                                n419 = call "Motors Status.vi"("error in"=w834, "VISA in"=w832, "Axis"=2, "Axis Multiplier"=w830) -> ("error out"=w833:errorcluster, "VISA out"=w831:refnum<visa-resource-name>, "OS"=w835:i32, "Actual Position (mm or deg)"=w827:dbl)  [unwired: 3 in]
                                n420 = property on="Y-Axis (mm)" class="DigNum (strict)"("Value"=w827) -> ()  [unwired: 2 in, 2 out]
                                n421 = call "Motors Decipher Status.vi"("OS"=w835) -> ("Status"=w826:string)
                                n422 = property on="Status Y" class="Str"("Value"=w826) -> ()  [unwired: 2 in, 2 out]
                                }
                                n423 = call "Motors Stop.vi"("error in"=w824, "Axis"=w816, "VISA in"=w825) -> ("error out"=w822:errorcluster, "VISA out"=w823:refnum<visa-resource-name>)
                                }
                              }
                            }
                            frame #1 {
                              n424 = property on="y+" class="Bool (strict)"("Value"=FALSE) -> ()  [unwired: 2 in, 2 out]
                              n425 = property on="y-" class="Bool (strict)"("Value"=FALSE) -> ()  [unwired: 2 in, 2 out]
                            }
                          }
                        }
                      }
                      n426 = case shown="False" w126 {
                        tunnel: w130 -> [w709 w715]
                        tunnel: w129 -> [w708 w714]
                        tunnel: [w709 w713] -> w124
                        tunnel: [w708 w712] -> w79
                        frame False {
                        }
                        frame True {
                          n427 = flat-sequence {
                            tunnel: w715 -> [w721]
                            tunnel: w714 -> [w720]
                            tunnel: [w719] -> w711
                            tunnel: [w718] -> w710
                            tunnel: [w775] -> w712
                            tunnel: [w776] -> w713
                            tunnel: w711 -> [w776]
                            tunnel: w710 -> [w775]
                            frame #0 {
                              n428 = property on="Z Multiplier" class="DigNum (strict)"() -> ("Value"=w716:u32)  [unwired: 2 in, 2 out]
                              n429 = property on="Jog-Mode" class="Bool (strict)"() -> ("Value"=w717:bool)  [unwired: 2 in, 2 out]
                              n430 = case shown="True" w717 {
                                tunnel: w721 -> [w727 w749]
                                tunnel: w720 -> [w726 w752]
                                tunnel: [w725 w754] -> w719
                                tunnel: [w724 w753] -> w718
                                tunnel: w716 -> [w723 w746]
                                frame False {
                                n431 = property on="Z Moving" class="Bool (strict)"() -> ("Value"=w722:bool)  [unwired: 2 in, 2 out]
                                n432 = case shown="False" w722 {
                                tunnel: w727 -> [w734 w743]
                                tunnel: w726 -> [w737 w742]
                                tunnel: [w735 w743] -> w725
                                tunnel: [w736 w742] -> w724
                                tunnel: w723 -> [w731 _]
                                frame False {
                                n433 = property on="Z Moving" class="Bool (strict)"("Value"=TRUE ("Y Moving")) -> ()  [unwired: 2 in, 2 out]
                                n434 = property on="z-" class="Bool (strict)"() -> ("Value"=w728:bool)  [unwired: 2 in, 2 out]
                                n435 = case shown="True" w728 {
                                tunnel: "Delta Z (mm)" -> [w738 w740]
                                tunnel: [w738 w739] -> w733
                                frame False {
                                }
                                frame True {
                                n436 = Multiply(x=w740, y=-1.0) -> (x*y=w739:dbl)
                                }
                                }
                                n437 = call "Motors Move Relative.vi"("Axis Multiplier"=w731, "Axis"=3, "error in"=w737, "VISA in"=w734, "Distance (mm)"=w733) -> ("error out"=w736:errorcluster, "VISA out"=w735:refnum<visa-resource-name>)  [unwired: 5 in]
                                }
                                frame True {
                                }
                                }
                                }
                                frame True {
                                w747 = 3 ("Axis")
                                n438 = property on="z-" class="Bool (strict)"() -> ("Value"=w744:bool)  [unwired: 2 in, 2 out]
                                n439 = case shown="True" w744 {
                                tunnel: "Z Speed (mm/s)" -> [w769 w771]
                                tunnel: [w769 w770] -> w750
                                frame False {
                                }
                                frame True {
                                n440 = Multiply(x=w771, y=-1.0) -> (x*y=w770:dbl)
                                }
                                }
                                n441 = call "Motors Move Constant Velocity.vi"("Axis Multiplier"=w746, "Axis"=w747, "error in"=w752, "VISA in"=w749, "Speed (mm/s)"=w750) -> ("error out"=w751:errorcluster, "VISA out"=w748:refnum<visa-resource-name>)  [unwired: 5 in]
                                n442 = while {
                                tunnel: w748 -> [w763]
                                tunnel: [w762] -> w756
                                tunnel: w751 -> [w765]
                                tunnel: [w764] -> w755
                                tunnel: w746 -> [w761]
                                stop <- w768 continue-if-true
                                n443 = property on="z+" class="Bool (strict)"() -> ("Value"=w760:bool)  [unwired: 2 in, 2 out]
                                n444 = property on="z-" class="Bool (strict)"() -> ("Value"=w759:bool)  [unwired: 2 in, 2 out]
                                n445 = Or(x=w760, y=w759) -> (x .or. y?=w768:bool)
                                n446 = call "Motors Status.vi"("error in"=w765, "VISA in"=w763, "Axis"=3, "Axis Multiplier"=w761) -> ("error out"=w764:errorcluster, "VISA out"=w762:refnum<visa-resource-name>, "OS"=w766:i32, "Actual Position (mm or deg)"=w758:dbl)  [unwired: 3 in]
                                n447 = call "Motors Decipher Status.vi"("OS"=w766) -> ("Status"=w757:string)
                                n448 = property on="Z-Axis (mm)" class="DigNum (strict)"("Value"=w758) -> ()  [unwired: 2 in, 2 out]
                                n449 = property on="Status Z" class="Str"("Value"=w757) -> ()  [unwired: 2 in, 2 out]
                                }
                                n450 = call "Motors Stop.vi"("error in"=w755, "Axis"=w747, "VISA in"=w756) -> ("error out"=w753:errorcluster, "VISA out"=w754:refnum<visa-resource-name>)
                                }
                              }
                            }
                            frame #1 {
                              n451 = property on="z+" class="Bool (strict)"("Value"=FALSE) -> ()  [unwired: 2 in, 2 out]
                              n452 = property on="z-" class="Bool (strict)"("Value"=FALSE) -> ()  [unwired: 2 in, 2 out]
                            }
                          }
                        }
                      }
                      n453 = case shown="True" w125 {
                        tunnel: w124 -> [w640 w646]
                        tunnel: w79 -> [w639 w645]
                        tunnel: [w640 w644] -> w116
                        tunnel: [w639 w643] -> w115
                        frame False {
                        }
                        frame True {
                          n454 = flat-sequence {
                            tunnel: w646 -> [w652]
                            tunnel: w645 -> [w651]
                            tunnel: [w650] -> w642
                            tunnel: [w649] -> w641
                            tunnel: [w706] -> w643
                            tunnel: [w707] -> w644
                            tunnel: w642 -> [w707]
                            tunnel: w641 -> [w706]
                            frame #0 {
                              n455 = property on="Theta Multiplier" class="DigNum (strict)"() -> ("Value"=w647:u32)  [unwired: 2 in, 2 out]
                              n456 = property on="Jog-Mode" class="Bool (strict)"() -> ("Value"=w648:bool)  [unwired: 2 in, 2 out]
                              n457 = case shown="False" w648 {
                                tunnel: w652 -> [w658 w680]
                                tunnel: w651 -> [w657 w683]
                                tunnel: [w656 w685] -> w650
                                tunnel: [w655 w684] -> w649
                                tunnel: w647 -> [w654 w677]
                                frame False {
                                n458 = property on="Theta Moving" class="Bool (strict)"() -> ("Value"=w653:bool)  [unwired: 2 in, 2 out]
                                n459 = case shown="False" w653 {
                                tunnel: w658 -> [w665 w674]
                                tunnel: w657 -> [w668 w673]
                                tunnel: [w666 w674] -> w656
                                tunnel: [w667 w673] -> w655
                                tunnel: w654 -> [w662 _]
                                frame False {
                                n460 = property on="Theta Moving" class="Bool (strict)"("Value"=TRUE ("Y Moving")) -> ()  [unwired: 2 in, 2 out]
                                n461 = property on="theta-" class="Bool (strict)"() -> ("Value"=w661:bool)  [unwired: 2 in, 2 out]
                                n462 = case shown="True" w661 {
                                tunnel: "Delta Theta (deg)" -> [w669 w671]
                                tunnel: [w669 w670] -> w664
                                frame False {
                                }
                                frame True {
                                n463 = Multiply(x=w671, y=-1.0) -> (x*y=w670:dbl)
                                }
                                }
                                n464 = call "Motors Move Relative.vi"("Axis Multiplier"=w662, "Axis"=4, "error in"=w668, "VISA in"=w665, "Distance (mm)"=w664) -> ("error out"=w667:errorcluster, "VISA out"=w666:refnum<visa-resource-name>)  [unwired: 5 in]
                                }
                                frame True {
                                }
                                }
                                }
                                frame True {
                                w678 = 4 ("Axis")
                                n465 = property on="theta-" class="Bool (strict)"() -> ("Value"=w676:bool)  [unwired: 2 in, 2 out]
                                n466 = case shown="True" w676 {
                                tunnel: "Theta Speed (deg/s)" -> [w700 w702]
                                tunnel: [w700 w701] -> w681
                                frame False {
                                }
                                frame True {
                                n467 = Multiply(x=w702, y=-1.0) -> (x*y=w701:dbl)
                                }
                                }
                                n468 = call "Motors Move Constant Velocity.vi"("Axis Multiplier"=w677, "Axis"=w678, "error in"=w683, "VISA in"=w680, "Speed (mm/s)"=w681) -> ("error out"=w682:errorcluster, "VISA out"=w679:refnum<visa-resource-name>)  [unwired: 5 in]
                                n469 = while {
                                tunnel: w679 -> [w694]
                                tunnel: [w693] -> w687
                                tunnel: w682 -> [w696]
                                tunnel: [w695] -> w686
                                tunnel: w677 -> [w692]
                                stop <- w699 continue-if-true
                                n470 = property on="theta-" class="Bool (strict)"() -> ("Value"=w691:bool)  [unwired: 2 in, 2 out]
                                n471 = property on="theta+" class="Bool (strict)"() -> ("Value"=w690:bool)  [unwired: 2 in, 2 out]
                                n472 = Or(x=w691, y=w690) -> (x .or. y?=w699:bool)
                                n473 = call "Motors Status.vi"("error in"=w696, "VISA in"=w694, "Axis"=4, "Axis Multiplier"=w692) -> ("error out"=w695:errorcluster, "VISA out"=w693:refnum<visa-resource-name>, "OS"=w697:i32, "Actual Position (mm or deg)"=w689:dbl)  [unwired: 3 in]
                                n474 = call "Motors Decipher Status.vi"("OS"=w697) -> ("Status"=w688:string)
                                n475 = property on="Theta (deg)" class="DigNum (strict)"("Value"=w689) -> ()  [unwired: 2 in, 2 out]
                                n476 = property on="Status Theta" class="Str"("Value"=w688) -> ()  [unwired: 2 in, 2 out]
                                }
                                n477 = call "Motors Stop.vi"("error in"=w686, "Axis"=w678, "VISA in"=w687) -> ("error out"=w684:errorcluster, "VISA out"=w685:refnum<visa-resource-name>)
                                }
                              }
                            }
                            frame #1 {
                              n478 = property on="theta+" class="Bool (strict)"("Value"=FALSE) -> ()  [unwired: 2 in, 2 out]
                              n479 = property on="theta-" class="Bool (strict)"("Value"=FALSE) -> ()  [unwired: 2 in, 2 out]
                            }
                          }
                        }
                      }
                      n480 = case shown="False" "X Set Slew Speed" {
                        tunnel: [w630 w634] -> w119
                        tunnel: w116 -> [w630 w635]
                        tunnel: [w629 w637] -> w121
                        tunnel: w115 -> [w629 w638]
                        frame False {
                        }
                        frame True {
                          # "Set motor's movement speed."
                          n481 = property on="Update Params" class="Bool (strict)"("Value"=TRUE ("Need to Update Motor Parameters")) -> ()  [unwired: 2 in, 2 out]
                          n482 = property on="X Multiplier" class="DigNum (strict)"() -> ("Value"=w632:u32)  [unwired: 2 in, 2 out]
                          n483 = call "Motors Move Speed.vi"("Speed (mm or degree/sec)"="User X Slew Speed", "error in"=w638, "VISA in"=w635, "Axis"=u32 1, "Axis Multiplier"=w632) -> ("error out"=w637:errorcluster, "VISA out"=w634:refnum<visa-resource-name>)  [unwired: 5 in]
                        }
                      }
                      n484 = case shown="False" "Y Set Slew Speed" {
                        tunnel: [w620 w625] -> w118
                        tunnel: w119 -> [w620 w624]
                        tunnel: [w619 w627] -> w78
                        tunnel: w121 -> [w619 w628]
                        frame False {
                        }
                        frame True {
                          n485 = property on="Update Params" class="Bool (strict)"("Value"=TRUE ("Need to Update Motor Parameters")) -> ()  [unwired: 2 in, 2 out]
                          n486 = property on="Y Multiplier" class="DigNum (strict)"() -> ("Value"=w622:u32)  [unwired: 2 in, 2 out]
                          n487 = call "Motors Move Speed.vi"("Speed (mm or degree/sec)"="User Y Slew Speed", "error in"=w628, "VISA in"=w624, "Axis"=u32 2, "Axis Multiplier"=w622) -> ("error out"=w627:errorcluster, "VISA out"=w625:refnum<visa-resource-name>)  [unwired: 5 in]
                        }
                      }
                      n488 = case shown="False" "Z Set Slew Speed" {
                        tunnel: [w610 w615] -> w117
                        tunnel: w118 -> [w610 w614]
                        tunnel: [w609 w617] -> w120
                        tunnel: w78 -> [w609 w618]
                        frame False {
                        }
                        frame True {
                          n489 = property on="Update Params" class="Bool (strict)"("Value"=TRUE ("Need to Update Motor Parameters")) -> ()  [unwired: 2 in, 2 out]
                          n490 = property on="Z Multiplier" class="DigNum (strict)"() -> ("Value"=w612:u32)  [unwired: 2 in, 2 out]
                          n491 = call "Motors Move Speed.vi"("Speed (mm or degree/sec)"="User Z Slew Speed", "error in"=w618, "VISA in"=w614, "Axis"=u32 3, "Axis Multiplier"=w612) -> ("error out"=w617:errorcluster, "VISA out"=w615:refnum<visa-resource-name>)  [unwired: 5 in]
                        }
                      }
                      n492 = case shown="False" "Theta Set Slew Speed" {
                        tunnel: [w600 w605] -> w109
                        tunnel: w117 -> [w600 w604]
                        tunnel: [w599 w606] -> w110
                        tunnel: w120 -> [w599 w608]
                        frame False {
                        }
                        frame True {
                          n493 = property on="Update Params" class="Bool (strict)"("Value"=TRUE ("Need to Update Motor Parameters")) -> ()  [unwired: 2 in, 2 out]
                          n494 = property on="Theta Multiplier" class="DigNum (strict)"() -> ("Value"=w602:u32)  [unwired: 2 in, 2 out]
                          n495 = call "Motors Move Speed.vi"("Speed (mm or degree/sec)"="User Theta Slew Speed", "error in"=w608, "VISA in"=w604, "Axis"=u32 4, "Axis Multiplier"=w602) -> ("error out"=w606:errorcluster, "VISA out"=w605:refnum<visa-resource-name>)  [unwired: 5 in]
                        }
                      }
                      n496 = case shown="0, Default" w86 {
                        tunnel: w110 -> [w373 w388 w402 w418]
                        tunnel: w109 -> [w374 w389 w404 w419]
                        tunnel: [w372 w386 w401 w417] -> w76
                        tunnel: [w371 w387 w403 w416] -> w77
                        frame 0, Default {
                          # "It takes too long to update every motor's position and status on every loop iteration.  Thus, we instead do only one motor/iteration."
                          n497 = property on="X Multiplier" class="DigNum (strict)"() -> ("Value"=w370:u32)  [unwired: 2 in, 2 out]
                          n498 = call "Motors Status.vi"("error in"=w373, "VISA in"=w374, "Axis"=1, "Axis Multiplier"=w370) -> ("error out"=w372:errorcluster, "VISA out"=w371:refnum<visa-resource-name>, "OS"=w377:i32, "Actual Position (mm or deg)"=w366:dbl)  [unwired: 3 in]
                          n499 = property on="X-Axis (mm)" class="DigNum (strict)"("Value"=w366) -> ()  [unwired: 2 in, 2 out]
                          n500 = call "Motors Decipher Status.vi"("OS"=w377) -> ("Status"=w369:string)
                          n501 = property on="Status X" class="Str"("Value"=w369) -> ()  [unwired: 2 in, 2 out]
                          n502 = property on="X (mm)" class="LVObjRef (strict)"() -> ("Value"=w367:refnum<vi>)  [unwired: 2 in, 2 out]
                          n503 = Equal?(x=w369, y="Idle") -> (x = y?=w375:bool)
                          n504 = case shown="True" w375 {
                            tunnel: [TRUE FALSE] -> w368
                            frame False {
                            }
                            frame True {
                            }
                          }
                          n505 = property class="DigNum (strict)"(reference=w367, "Value"=w366) -> ()  [unwired: 1 in, 2 out]
                          n506 = property on="X Moving" class="Bool (strict)"("Value"=w368) -> ()  [unwired: 2 in, 2 out]
                        }
                        frame 1 {
                          n507 = property on="Y Multiplier" class="DigNum (strict)"() -> ("Value"=w385:u32)  [unwired: 2 in, 2 out]
                          n508 = call "Motors Status.vi"("error in"=w388, "VISA in"=w389, "Axis"=2, "Axis Multiplier"=w385) -> ("error out"=w386:errorcluster, "VISA out"=w387:refnum<visa-resource-name>, "OS"=w392:i32, "Actual Position (mm or deg)"=w381:dbl)  [unwired: 3 in]
                          n509 = property on="Y-Axis (mm)" class="DigNum (strict)"("Value"=w381) -> ()  [unwired: 2 in, 2 out]
                          n510 = call "Motors Decipher Status.vi"("OS"=w392) -> ("Status"=w384:string)
                          n511 = property on="Status Y" class="Str"("Value"=w384) -> ()  [unwired: 2 in, 2 out]
                          n512 = property on="Y (mm)" class="LVObjRef (strict)"() -> ("Value"=w382:refnum<vi>)  [unwired: 2 in, 2 out]
                          n513 = Equal?(x=w384, y="Idle") -> (x = y?=w390:bool)
                          n514 = case shown="False" w390 {
                            tunnel: [TRUE FALSE] -> w383
                            frame False {
                            }
                            frame True {
                            }
                          }
                          n515 = property class="DigNum (strict)"(reference=w382, "Value"=w381) -> ()  [unwired: 1 in, 2 out]
                          n516 = property on="Y Moving" class="Bool (strict)"("Value"=w383) -> ()  [unwired: 2 in, 2 out]
                        }
                        frame 2 {
                          n517 = property on="Z Multiplier" class="DigNum (strict)"() -> ("Value"=w400:u32)  [unwired: 2 in, 2 out]
                          n518 = call "Motors Status.vi"("error in"=w402, "VISA in"=w404, "Axis"=3, "Axis Multiplier"=w400) -> ("error out"=w401:errorcluster, "VISA out"=w403:refnum<visa-resource-name>, "OS"=w407:i32, "Actual Position (mm or deg)"=w396:dbl)  [unwired: 3 in]
                          n519 = property on="Z-Axis (mm)" class="DigNum (strict)"("Value"=w396) -> ()  [unwired: 2 in, 2 out]
                          n520 = call "Motors Decipher Status.vi"("OS"=w407) -> ("Status"=w399:string)
                          n521 = property on="Status Z" class="Str"("Value"=w399) -> ()  [unwired: 2 in, 2 out]
                          n522 = property on="Z (mm)" class="LVObjRef (strict)"() -> ("Value"=w397:refnum<vi>)  [unwired: 2 in, 2 out]
                          n523 = Equal?(x=w399, y="Idle") -> (x = y?=w405:bool)
                          n524 = property class="DigNum (strict)"(reference=w397, "Value"=w396) -> ()  [unwired: 1 in, 2 out]
                          n525 = case shown="True" w405 {
                            tunnel: [TRUE FALSE] -> w398
                            frame False {
                            }
                            frame True {
                            }
                          }
                          n526 = property on="Z Moving" class="Bool (strict)"("Value"=w398) -> ()  [unwired: 2 in, 2 out]
                        }
                        frame 3 {
                          n527 = property on="Theta Multiplier" class="DigNum (strict)"() -> ("Value"=w415:u32)  [unwired: 2 in, 2 out]
                          n528 = call "Motors Status.vi"("error in"=w418, "VISA in"=w419, "Axis"=4, "Axis Multiplier"=w415) -> ("error out"=w417:errorcluster, "VISA out"=w416:refnum<visa-resource-name>, "OS"=w422:i32, "Actual Position (mm or deg)"=w411:dbl)  [unwired: 3 in]
                          n529 = property on="Theta (deg)" class="LVObjRef (strict)"() -> ("Value"=w412:refnum<vi>)  [unwired: 2 in, 2 out]
                          n530 = property on="Theta (deg)" class="DigNum (strict)"("Value"=w411) -> ()  [unwired: 2 in, 2 out]
                          n531 = property class="DigNum (strict)"(reference=w412, "Value"=w411) -> ()  [unwired: 1 in, 2 out]
                          n532 = call "Motors Decipher Status.vi"("OS"=w422) -> ("Status"=w413:string)
                          n533 = property on="Status Theta" class="Str"("Value"=w413) -> ()  [unwired: 2 in, 2 out]
                          n534 = Equal?(x=w413, y="Idle") -> (x = y?=w420:bool)
                          n535 = case shown="False" w420 {
                            tunnel: [TRUE FALSE] -> w414
                            frame False {
                            }
                            frame True {
                            }
                          }
                          n536 = property on="Theta Moving" class="Bool (strict)"("Value"=w414) -> ()  [unwired: 2 in, 2 out]
                        }
                      }
                      n537 = case shown="False" "Go To Saved Position" {
                        tunnel: w76 -> [w568 w576]
                        tunnel: w77 -> [w567 w577]
                        tunnel: [w568 w590] -> w107
                        tunnel: [w567 w589] -> w106
                        frame False {
                        }
                        frame True {
                          w587 = 4 ("index (row)")
                          w585 = 3 ("index (row)")
                          w582 = 2 ("index (row)")
                          w579 = 1 ("index (row)")
                          # "Move to one of the positions in the list."
                          n538 = call "Motors Position Load.vi"("error in"=w576, "file path"="Saved Positions") -> ("error out"=w575:errorcluster, "Positions"=w593:string[][])
                          n539 = Index Array(array=w593, index (row)=w587, index (col)="Defined Positions") -> (element=w594:string)
                          n540 = Index Array(array=w593, index (row)=w585, index (col)="Defined Positions") -> (element=w595:string)
                          n541 = Index Array(array=w593, index (row)=w582, index (col)="Defined Positions") -> (element=w597:string)
                          n542 = Index Array(array=w593, index (row)=w579, index (col)="Defined Positions") -> (element=w598:string)
                          n543 = property on="X Multiplier" class="DigNum (strict)"() -> ("Value"=w574:u32)  [unwired: 2 in, 2 out]
                          n544 = Fract/Exp String To Number(string=w594) -> (number=w588:dbl)  [unwired: 3 in, 1 out]
                          n545 = Fract/Exp String To Number(string=w595) -> (number=w584:dbl)  [unwired: 3 in, 1 out]
                          n546 = Fract/Exp String To Number(string=w597) -> (number=w581:dbl)  [unwired: 3 in, 1 out]
                          n547 = Fract/Exp String To Number(string=w598) -> (number=w578:dbl)  [unwired: 3 in, 1 out]
                          n548 = property on="Y Multiplier" class="DigNum (strict)"() -> ("Value"=w573:u32)  [unwired: 2 in, 2 out]
                          n549 = call "Motors Move Absolute.vi"("Axis Multiplier"=w574, "Axis"=w579, "error in"=w575, "VISA in"=w577, "Position (mm or degree)"=w578) -> ("error out"=w596:errorcluster, "VISA out"=w580:refnum<visa-resource-name>)  [unwired: 5 in]
                          n550 = property on="Z Multiplier" class="DigNum (strict)"() -> ("Value"=w572:u32)  [unwired: 2 in, 2 out]
                          n551 = call "Motors Move Absolute.vi"("Axis Multiplier"=w573, "Axis"=w582, "error in"=w596, "VISA in"=w580, "Position (mm or degree)"=w581) -> ("error out"=w592:errorcluster, "VISA out"=w583:refnum<visa-resource-name>)  [unwired: 5 in]
                          n552 = property on="Theta Multiplier" class="DigNum (strict)"() -> ("Value"=w571:u32)  [unwired: 2 in, 2 out]
                          n553 = call "Motors Move Absolute.vi"("Axis Multiplier"=w572, "Axis"=w585, "error in"=w592, "VISA in"=w583, "Position (mm or degree)"=w584) -> ("error out"=w591:errorcluster, "VISA out"=w586:refnum<visa-resource-name>)  [unwired: 5 in]
                          n554 = call "Motors Move Absolute.vi"("Axis Multiplier"=w571, "Axis"=w587, "error in"=w591, "VISA in"=w586, "Position (mm or degree)"=w588) -> ("error out"=w590:errorcluster, "VISA out"=w589:refnum<visa-resource-name>)  [unwired: 5 in]
                        }
                      }
                      n555 = case shown="True" w105 {
                        tunnel: w107 -> [w501 w504]
                        tunnel: w106 -> [w500 w505]
                        tunnel: [w500 w503] -> w73
                        tunnel: [w501 w502] -> w71
                        frame False {
                        }
                        frame True {
                          # "It takes a very long time to update all of the motor's parameters.  Thus, we only do it when a motor operation calls for it (see for example, Set Slew Speed)."
                          n556 = flat-sequence {
                            tunnel: w505 -> [w543]
                            tunnel: w504 -> [w542]
                            tunnel: [w541] -> w503
                            tunnel: [w540] -> w502
                            frame #0 {
                              # "Deactivate mouse and set status message."
                              n557 = property on="Motors Status" class="Str"("Value"="Updating Motor Parameters\nThis Should Take About 5 Seconds" ("Status Theta")) -> ()  [unwired: 2 in, 2 out]
                            }
                            frame #1 {
                              # "Query the values of all parameters from each motor, extract the important information, and update the indicators."
                              n558 = call "Motors Status Verbose.vi"("Axis"=1, "VISA in"=w543, "error in"=w542) -> ("Slew Speed (mm or deg/s)"=→"X Slew Speed":dbl, "Jogger Normal Speed (mm or deg/s)"=→"X Jogger Normal Speed":dbl, "Jogger Fast Speed (mm or deg/s)"=→"X Jogger Fast Speed":dbl, "Actual Position (mm or deg)"=w510:dbl, "OS"=w550:i32, "Mode"=→"X Action":string, "VISA out"=w559:refnum<visa-resource-name>, "Creep Speed (mm or deg/s)"=w537:dbl, "error out"=w547:errorcluster)  [unwired: 4 in]
                              n559 = property on="Z (mm)" class="LVObjRef (strict)"() -> ("Value"=w513:refnum<vi>)  [unwired: 2 in, 2 out]
                              n560 = property on="X (mm)" class="LVObjRef (strict)"() -> ("Value"=w511:refnum<vi>)  [unwired: 2 in, 2 out]
                              n561 = property on="Y (mm)" class="LVObjRef (strict)"() -> ("Value"=w512:refnum<vi>)  [unwired: 2 in, 2 out]
                              n562 = property on="Theta (deg)" class="LVObjRef (strict)"() -> ("Value"=w514:refnum<vi>)  [unwired: 2 in, 2 out]
                              n563 = property class="DigNum (strict)"(reference=w511, "Value"=w510) -> ()  [unwired: 1 in, 2 out]
                              n564 = property on="X-Axis (mm)" class="DigNum (strict)"("Value"=w510) -> ()  [unwired: 2 in, 2 out]
                              n565 = call "Motors Decipher Status.vi"("OS"=w550) -> ("Status"=w522:string)
                              n566 = call "Motors Status Verbose.vi"("Axis"=2, "VISA in"=w559, "error in"=w547) -> ("Slew Speed (mm or deg/s)"=→"Y Slew Speed":dbl, "Jogger Normal Speed (mm or deg/s)"=→"Y Jogger Normal Speed":dbl, "Jogger Fast Speed (mm or deg/s)"=→"Y Jogger Fast Speed":dbl, "Actual Position (mm or deg)"=w509:dbl, "OS"=w551:i32, "Mode"=→"Y Action":string, "VISA out"=w560:refnum<visa-resource-name>, "Creep Speed (mm or deg/s)"=w535:dbl, "error out"=w548:errorcluster)  [unwired: 4 in]
                              n567 = property class="DigNum (strict)"(reference=w512, "Value"=w509) -> ()  [unwired: 1 in, 2 out]
                              n568 = property on="User X Slew Speed" class="DigNum (strict)"("Minimum"=w537) -> ()  [unwired: 2 in, 2 out]
                              n569 = property on="Status X" class="Str"("Value"=w522) -> ()  [unwired: 2 in, 2 out]
                              n570 = property on="Y-Axis (mm)" class="DigNum (strict)"("Value"=w509) -> ()  [unwired: 2 in, 2 out]
                              n571 = call "Motors Decipher Status.vi"("OS"=w551) -> ("Status"=w521:string)
                              n572 = call "Motors Status Verbose.vi"("Axis"=3, "VISA in"=w560, "error in"=w548) -> ("Slew Speed (mm or deg/s)"=→"Z Slew Speed":dbl, "Jogger Normal Speed (mm or deg/s)"=→"Z Jogger Normal Speed":dbl, "Jogger Fast Speed (mm or deg/s)"=→"Z Jogger Fast Speed":dbl, "Actual Position (mm or deg)"=w508:dbl, "OS"=w552:i32, "Mode"=→"Z Action":string, "VISA out"=w561:refnum<visa-resource-name>, "Creep Speed (mm or deg/s)"=w533:dbl, "error out"=w549:errorcluster)  [unwired: 4 in]
                              n573 = property class="DigNum (strict)"(reference=w513, "Value"=w508) -> ()  [unwired: 1 in, 2 out]
                              n574 = property on="User Y Slew Speed" class="DigNum (strict)"("Minimum"=w535) -> ()  [unwired: 2 in, 2 out]
                              n575 = Not Equal?(x=w522, y="Idle") -> (x != y?=w518:bool)
                              n576 = property on="Status Y" class="Str"("Value"=w521) -> ()  [unwired: 2 in, 2 out]
                              n577 = property on="X Moving" class="Bool (strict)"("Value"=w518) -> ()  [unwired: 2 in, 2 out]
                              n578 = property on="Z-Axis (mm)" class="DigNum (strict)"("Value"=w508) -> ()  [unwired: 2 in, 2 out]
                              n579 = property on="User Z Slew Speed" class="DigNum (strict)"("Minimum"=w533) -> ()  [unwired: 2 in, 2 out]
                              n580 = call "Motors Status Verbose.vi"("Axis"=4, "VISA in"=w561, "error in"=w549) -> ("Slew Speed (mm or deg/s)"=→"Theta Slew Speed":dbl, "Jogger Normal Speed (mm or deg/s)"=→"Theta Jogger Normal Speed":dbl, "Jogger Fast Speed (mm or deg/s)"=→"Theta Jogger Fast Speed":dbl, "Actual Position (mm or deg)"=w507:dbl, "OS"=w553:i32, "Mode"=→"Theta Action":string, "VISA out"=w541:refnum<visa-resource-name>, "Creep Speed (mm or deg/s)"=w531:dbl, "error out"=w540:errorcluster)  [unwired: 4 in]
                              n581 = property class="DigNum (strict)"(reference=w514, "Value"=w507) -> ()  [unwired: 1 in, 2 out]
                              n582 = call "Motors Decipher Status.vi"("OS"=w552) -> ("Status"=w520:string)
                              n583 = Not Equal?(x=w521, y="Idle") -> (x != y?=w517:bool)
                              n584 = property on="Status Z" class="Str"("Value"=w520) -> ()  [unwired: 2 in, 2 out]
                              n585 = property on="Theta (deg)" class="DigNum (strict)"("Value"=w507) -> ()  [unwired: 2 in, 2 out]
                              n586 = property on="User Theta Slew Speed" class="DigNum (strict)"("Minimum"=w531) -> ()  [unwired: 2 in, 2 out]
                              n587 = call "Motors Decipher Status.vi"("OS"=w553) -> ("Status"=w519:string)
                              n588 = property on="Y Moving" class="Bool (strict)"("Value"=w517) -> ()  [unwired: 2 in, 2 out]
                              n589 = property on="Status Theta" class="Str"("Value"=w519) -> ()  [unwired: 2 in, 2 out]
                              n590 = Not Equal?(x=w520, y="Idle") -> (x != y?=w516:bool)
                              n591 = Not Equal?(x=w519, y="Idle") -> (x != y?=w515:bool)
                              n592 = property on="Z Moving" class="Bool (strict)"("Value"=w516) -> ()  [unwired: 2 in, 2 out]
                              n593 = property on="Theta Moving" class="Bool (strict)"("Value"=w515) -> ()  [unwired: 2 in, 2 out]
                            }
                            frame #2 {
                              # "Reactivate mouse and reset status message."
                              n594 = property on="Update Params" class="Bool (strict)"("Value"=FALSE ("Need to Update Motor Parameters")) -> ()  [unwired: 2 in, 2 out]
                              n595 = property on="Motors Status" class="Str"("Value"="Running" ("Status Theta")) -> ()  [unwired: 2 in, 2 out]
                            }
                          }
                        }
                      }
                      n596 = case shown="True" w85 {
                        tunnel: [w185 w191] -> w72
                        tunnel: w73 -> [w185 w193]
                        tunnel: w71 -> [w186 w192]
                        tunnel: [w186 w190] -> w70
                        frame False {
                        }
                        frame True {
                          n597 = flat-sequence {
                            tunnel: [w196] -> w188
                            tunnel: [w195] -> w187
                            tunnel: w193 -> [w197]
                            tunnel: w192 -> [w194]
                            tunnel: w188 -> [w297]
                            tunnel: w187 -> [w294]
                            tunnel: [w295] -> w190
                            tunnel: [w296] -> w189
                            tunnel: [w365] -> w191
                            tunnel: w189 -> [w365]
                            frame #0 {
                              n598 = case shown="No Error" w194 {
                                selector: w194 -> [w198 w292]
                                tunnel: w197 -> [w201 w293]
                                tunnel: [w200 w293] -> w196
                                tunnel: [w199 w292] -> w195
                                frame No Error {
                                n599 = while {
                                tunnel: w201 -> [w279]
                                tunnel: w198 -> [w275]
                                tunnel: [w271] -> w200
                                tunnel: [w270] -> w199
                                stop <- w233 stop-if-true
                                # "Quit if a motor is moving OR the position of motor # is already at <# Go To>\nOR the scan is no longer in progress (user pressed Abort)."
                                # "Wait until at least one motor starts moving."
                                n600 = property on="Y Go To" class="DigNum (strict)"() -> ("Value"=w251:dbl)  [unwired: 2 in, 2 out]
                                n601 = property on="X Go To" class="DigNum (strict)"() -> ("Value"=w265:dbl)  [unwired: 2 in, 2 out]
                                n602 = property on="Z Go To" class="DigNum (strict)"() -> ("Value"=w248:dbl)  [unwired: 2 in, 2 out]
                                n603 = property on="Theta Go To" class="DigNum (strict)"() -> ("Value"=w247:dbl)  [unwired: 2 in, 2 out]
                                n604 = property on="Scan in Progress" class="LVObjRef (strict)"() -> ("Value"=w231:refnum<vi>)  [unwired: 2 in, 2 out]
                                n605 = property class="Bool (strict)"(reference=w231) -> ("Value"=w230:bool)  [unwired: 1 in, 2 out]
                                n606 = property on="X Go?" class="Bool (strict)"() -> ("Value"=w227:bool)  [unwired: 2 in, 2 out]
                                n607 = property on="Theta Go?" class="Bool (strict)"() -> ("Value"=w224:bool)  [unwired: 2 in, 2 out]
                                n608 = property on="Y Go?" class="Bool (strict)"() -> ("Value"=w226:bool)  [unwired: 2 in, 2 out]
                                n609 = property on="Z Go?" class="Bool (strict)"() -> ("Value"=w225:bool)  [unwired: 2 in, 2 out]
                                n610 = Not(x=w230) -> (.not. x?=w229:bool)
                                n611 = Compound Arithmetic op=OR(w227, w226, w225, w224) -> (invert w223:bool)
                                n612 = property on="X Multiplier" class="DigNum (strict)"() -> ("Value"=w261:u32)  [unwired: 2 in, 2 out]
                                n613 = Reciprocal(x=w261) -> (1/x=w260:dbl)
                                n614 = property on="Y Multiplier" class="DigNum (strict)"() -> ("Value"=w249:u32)  [unwired: 2 in, 2 out]
                                n615 = Reciprocal(x=w249) -> (1/x=w259:dbl)
                                n616 = call "Motors Status.vi"("error in"=w275, "VISA in"=w279, "Axis"=1, "Axis Multiplier"=w261) -> ("error out"=w274:errorcluster, "VISA out"=w278:refnum<visa-resource-name>, "OS"=w281:i32, "Actual Position (mm or deg)"=w264:dbl)  [unwired: 3 in]
                                n617 = Subtract(x=w265, y=w264) -> (x-y=w263:dbl)
                                n618 = Absolute Value(x=w263) -> (abs(x)=w262:dbl)
                                n619 = Less Or Equal?(x=w262, y=w260) -> (x <= y?=w242:bool)
                                n620 = And(x=w227, y=w242) -> (x .and. y?=w238:bool)
                                n621 = property on="X-Axis (mm)" class="DigNum (strict)"("Value"=w264) -> ()  [unwired: 2 in, 2 out]
                                n622 = call "Motors Decipher Status.vi"("OS"=w281) -> ("Status"=w220:string)
                                n623 = property on="Status X" class="Str"("Value"=w220) -> ()  [unwired: 2 in, 2 out]
                                n624 = property on="Z Multiplier" class="DigNum (strict)"() -> ("Value"=w244:u32)  [unwired: 2 in, 2 out]
                                n625 = Reciprocal(x=w244) -> (1/x=w255:dbl)
                                n626 = call "Motors Status.vi"("error in"=w274, "VISA in"=w278, "Axis"=2, "Axis Multiplier"=w249) -> ("error out"=w273:errorcluster, "VISA out"=w277:refnum<visa-resource-name>, "OS"=w284:i32, "Actual Position (mm or deg)"=w250:dbl)  [unwired: 3 in]
                                n627 = Subtract(x=w251, y=w250) -> (x-y=w257:dbl)
                                n628 = Absolute Value(x=w257) -> (abs(x)=w258:dbl)
                                n629 = Less Or Equal?(x=w258, y=w259) -> (x <= y?=w241:bool)
                                n630 = And(x=w226, y=w241) -> (x .and. y?=w237:bool)
                                n631 = property on="Y-Axis (mm)" class="DigNum (strict)"("Value"=w250) -> ()  [unwired: 2 in, 2 out]
                                n632 = call "Motors Decipher Status.vi"("OS"=w284) -> ("Status"=w216:string)
                                n633 = Not Equal?(x=w220, y="Idle") -> (x != y?=w218:bool)
                                n634 = Not Equal?(x=w220, y="Error") -> (x != y?=w221:bool)
                                n635 = property on="Status Y" class="Str"("Value"=w216) -> ()  [unwired: 2 in, 2 out]
                                n636 = call "Motors Status.vi"("error in"=w273, "VISA in"=w277, "Axis"=3, "Axis Multiplier"=w244) -> ("error out"=w272:errorcluster, "VISA out"=w276:refnum<visa-resource-name>, "OS"=w287:i32, "Actual Position (mm or deg)"=w246:dbl)  [unwired: 3 in]
                                n637 = Subtract(x=w248, y=w246) -> (x-y=w256:dbl)
                                n638 = Absolute Value(x=w256) -> (abs(x)=w254:dbl)
                                n639 = Less Or Equal?(x=w254, y=w255) -> (x <= y?=w240:bool)
                                n640 = And(x=w225, y=w240) -> (x .and. y?=w236:bool)
                                n641 = property on="Theta Multiplier" class="DigNum (strict)"() -> ("Value"=w243:u32)  [unwired: 2 in, 2 out]
                                n642 = Reciprocal(x=w243) -> (1/x=w253:dbl)
                                n643 = And(x=w221, y=w218) -> (x .and. y?=w217:bool)
                                n644 = property on="X Moving" class="Bool (strict)"("Value"=w217) -> ()  [unwired: 2 in, 2 out]
                                n645 = property on="Z-Axis (mm)" class="DigNum (strict)"("Value"=w246) -> ()  [unwired: 2 in, 2 out]
                                n646 = call "Motors Decipher Status.vi"("OS"=w287) -> ("Status"=w211:string)
                                n647 = Not Equal?(x=w216, y="Idle") -> (x != y?=w214:bool)
                                n648 = property on="Status Z" class="Str"("Value"=w211) -> ()  [unwired: 2 in, 2 out]
                                n649 = call "Motors Status.vi"("error in"=w272, "VISA in"=w276, "Axis"=4, "Axis Multiplier"=w243) -> ("error out"=w270:errorcluster, "VISA out"=w271:refnum<visa-resource-name>, "OS"=w290:i32, "Actual Position (mm or deg)"=w245:dbl)  [unwired: 3 in]
                                n650 = Subtract(x=w247, y=w245) -> (x-y=w252:dbl)
                                n651 = Absolute Value(x=w252) -> (abs(x)=w232:dbl)
                                n652 = Less Or Equal?(x=w232, y=w253) -> (x <= y?=w239:bool)
                                n653 = And(x=w239, y=w224) -> (x .and. y?=w235:bool)
                                n654 = Compound Arithmetic op=OR(w238, w237, w236, w235) -> (w228:bool)
                                n655 = Or(x=w223, y=w228) -> (x .or. y?=w222:bool)
                                n656 = property on="Z (mm)" class="LVObjRef (strict)"() -> ("Value"=w267:refnum<vi>)  [unwired: 2 in, 2 out]
                                n657 = Not Equal?(x=w216, y="Error") -> (x != y?=w213:bool)
                                n658 = property on="X (mm)" class="LVObjRef (strict)"() -> ("Value"=w269:refnum<vi>)  [unwired: 2 in, 2 out]
                                n659 = property on="Y (mm)" class="LVObjRef (strict)"() -> ("Value"=w268:refnum<vi>)  [unwired: 2 in, 2 out]
                                n660 = property on="Theta (deg)" class="LVObjRef (strict)"() -> ("Value"=w266:refnum<vi>)  [unwired: 2 in, 2 out]
                                n661 = And(x=w213, y=w214) -> (x .and. y?=w212:bool)
                                n662 = property on="Y Moving" class="Bool (strict)"("Value"=w212) -> ()  [unwired: 2 in, 2 out]
                                n663 = property on="Theta (deg)" class="DigNum (strict)"("Value"=w245) -> ()  [unwired: 2 in, 2 out]
                                n664 = call "Motors Decipher Status.vi"("OS"=w290) -> ("Status"=w204:string)
                                n665 = Not Equal?(x=w211, y="Idle") -> (x != y?=w209:bool)
                                n666 = property class="DigNum (strict)"(reference=w269, "Value"=w264) -> ()  [unwired: 1 in, 2 out]
                                n667 = property class="DigNum (strict)"(reference=w268, "Value"=w250) -> ()  [unwired: 1 in, 2 out]
                                n668 = property class="DigNum (strict)"(reference=w267, "Value"=w246) -> ()  [unwired: 1 in, 2 out]
                                n669 = Not Equal?(x=w211, y="Error") -> (x != y?=w208:bool)
                                n670 = property class="DigNum (strict)"(reference=w266, "Value"=w245) -> ()  [unwired: 1 in, 2 out]
                                n671 = property on="Status Theta" class="Str"("Value"=w204) -> ()  [unwired: 2 in, 2 out]
                                n672 = And(x=w208, y=w209) -> (x .and. y?=w207:bool)
                                n673 = Not Equal?(x=w204, y="Error") -> (x != y?=w205:bool)
                                n674 = Not Equal?(x=w204, y="Idle") -> (x != y?=w206:bool)
                                n675 = property on="Z Moving" class="Bool (strict)"("Value"=w207) -> ()  [unwired: 2 in, 2 out]
                                n676 = And(x=w205, y=w206) -> (x .and. y?=w202:bool)
                                n677 = property on="Theta Moving" class="Bool (strict)"("Value"=w202) -> ()  [unwired: 2 in, 2 out]
                                n678 = Compound Arithmetic op=OR(w217, w212, w207, w202) -> (w234:bool)
                                n679 = Compound Arithmetic op=OR(w229, w222, w234) -> (w233:bool)
                                }
                                }
                                frame Error {
                                }
                              }
                            }
                            frame #1 {
                              n680 = case shown="No Error" w294 {
                                selector: w294 -> [w298 w348]
                                tunnel: w297 -> [w301 w349]
                                tunnel: [w300 w349] -> w296
                                tunnel: [w299 w348] -> w295
                                frame No Error {
                                n681 = while {
                                tunnel: w301 -> [w328]
                                tunnel: w298 -> [w324]
                                tunnel: [w315] -> w300
                                tunnel: [w314] -> w299
                                stop <- w303 continue-if-true
                                # "Keep going while at least one motor is moving\nAND the scan is still in progress."
                                # "Wait until all the motors stop moving.  Also, update the positions continuously in the meantime."
                                n682 = property on="Scan in Progress" class="LVObjRef (strict)"() -> ("Value"=w305:refnum<vi>)  [unwired: 2 in, 2 out]
                                n683 = property on="X Multiplier" class="DigNum (strict)"() -> ("Value"=w330:u32)  [unwired: 2 in, 2 out]
                                n684 = property class="Bool (strict)"(reference=w305) -> ("Value"=w302:bool)  [unwired: 1 in, 2 out]
                                n685 = property on="Y Multiplier" class="DigNum (strict)"() -> ("Value"=w335:u32)  [unwired: 2 in, 2 out]
                                n686 = call "Motors Status.vi"("error in"=w324, "VISA in"=w328, "Axis"=1, "Axis Multiplier"=w330) -> ("error out"=w323:errorcluster, "VISA out"=w327:refnum<visa-resource-name>, "OS"=w332:i32, "Actual Position (mm or deg)"=w309:dbl)  [unwired: 3 in]
                                n687 = property on="X-Axis (mm)" class="DigNum (strict)"("Value"=w309) -> ()  [unwired: 2 in, 2 out]
                                n688 = call "Motors Decipher Status.vi"("OS"=w332) -> ("Status"=w329:string)
                                n689 = property on="Status X" class="Str"("Value"=w329) -> ()  [unwired: 2 in, 2 out]
                                n690 = property on="Z Multiplier" class="DigNum (strict)"() -> ("Value"=w339:u32)  [unwired: 2 in, 2 out]
                                n691 = call "Motors Status.vi"("error in"=w323, "VISA in"=w327, "Axis"=2, "Axis Multiplier"=w335) -> ("error out"=w322:errorcluster, "VISA out"=w326:refnum<visa-resource-name>, "OS"=w337:i32, "Actual Position (mm or deg)"=w308:dbl)  [unwired: 3 in]
                                n692 = property on="Y-Axis (mm)" class="DigNum (strict)"("Value"=w308) -> ()  [unwired: 2 in, 2 out]
                                n693 = call "Motors Decipher Status.vi"("OS"=w337) -> ("Status"=w334:string)
                                n694 = Not Equal?(x=w329, y="Idle") -> (x != y?=w319:bool)
                                n695 = property on="Status Y" class="Str"("Value"=w334) -> ()  [unwired: 2 in, 2 out]
                                n696 = call "Motors Status.vi"("error in"=w322, "VISA in"=w326, "Axis"=3, "Axis Multiplier"=w339) -> ("error out"=w321:errorcluster, "VISA out"=w325:refnum<visa-resource-name>, "OS"=w341:i32, "Actual Position (mm or deg)"=w307:dbl)  [unwired: 3 in]
                                n697 = property on="Theta Multiplier" class="DigNum (strict)"() -> ("Value"=w344:u32)  [unwired: 2 in, 2 out]
                                n698 = property on="X Moving" class="Bool (strict)"("Value"=w319) -> ()  [unwired: 2 in, 2 out]
                                n699 = property on="Z-Axis (mm)" class="DigNum (strict)"("Value"=w307) -> ()  [unwired: 2 in, 2 out]
                                n700 = call "Motors Decipher Status.vi"("OS"=w341) -> ("Status"=w320:string)
                                n701 = Not Equal?(x=w334, y="Idle") -> (x != y?=w318:bool)
                                n702 = property on="Z (mm)" class="LVObjRef (strict)"() -> ("Value"=w311:refnum<vi>)  [unwired: 2 in, 2 out]
                                n703 = property on="X (mm)" class="LVObjRef (strict)"() -> ("Value"=w313:refnum<vi>)  [unwired: 2 in, 2 out]
                                n704 = property on="Y (mm)" class="LVObjRef (strict)"() -> ("Value"=w312:refnum<vi>)  [unwired: 2 in, 2 out]
                                n705 = property on="Theta (deg)" class="LVObjRef (strict)"() -> ("Value"=w310:refnum<vi>)  [unwired: 2 in, 2 out]
                                n706 = property on="Status Z" class="Str"("Value"=w320) -> ()  [unwired: 2 in, 2 out]
                                n707 = call "Motors Status.vi"("error in"=w321, "VISA in"=w325, "Axis"=4, "Axis Multiplier"=w344) -> ("error out"=w314:errorcluster, "VISA out"=w315:refnum<visa-resource-name>, "OS"=w346:i32, "Actual Position (mm or deg)"=w306:dbl)  [unwired: 3 in]
                                n708 = property on="Y Moving" class="Bool (strict)"("Value"=w318) -> ()  [unwired: 2 in, 2 out]
                                n709 = property on="Theta (deg)" class="DigNum (strict)"("Value"=w306) -> ()  [unwired: 2 in, 2 out]
                                n710 = property class="DigNum (strict)"(reference=w313, "Value"=w309) -> ()  [unwired: 1 in, 2 out]
                                n711 = call "Motors Decipher Status.vi"("OS"=w346) -> ("Status"=w343:string)
                                n712 = property class="DigNum (strict)"(reference=w312, "Value"=w308) -> ()  [unwired: 1 in, 2 out]
                                n713 = property class="DigNum (strict)"(reference=w311, "Value"=w307) -> ()  [unwired: 1 in, 2 out]
                                n714 = Not Equal?(x=w320, y="Idle") -> (x != y?=w317:bool)
                                n715 = property class="DigNum (strict)"(reference=w310, "Value"=w306) -> ()  [unwired: 1 in, 2 out]
                                n716 = property on="Status Theta" class="Str"("Value"=w343) -> ()  [unwired: 2 in, 2 out]
                                n717 = Not Equal?(x=w343, y="Idle") -> (x != y?=w316:bool)
                                n718 = property on="Z Moving" class="Bool (strict)"("Value"=w317) -> ()  [unwired: 2 in, 2 out]
                                n719 = property on="Theta Moving" class="Bool (strict)"("Value"=w316) -> ()  [unwired: 2 in, 2 out]
                                n720 = Compound Arithmetic op=OR(w319, w318, w317, w316) -> (w304:bool)
                                n721 = And(x=w302, y=w304) -> (x .and. y?=w303:bool)
                                }
                                }
                                frame Error {
                                }
                              }
                            }
                            frame #2 {
                              # "Set both the global <Set> and the local <Set?> to False to indicate that the motors have moved to their next position in the scan."
                              n722 = property on="Set" class="LVObjRef (strict)"() -> ("Value"=w363:refnum<vi>)  [unwired: 2 in, 2 out]
                              n723 = property on="Y Go?" class="Bool (strict)"("Value"=FALSE ("Y Go?")) -> ()  [unwired: 2 in, 2 out]
                              n724 = property on="Z Go?" class="Bool (strict)"("Value"=FALSE ("Z Go?")) -> ()  [unwired: 2 in, 2 out]
                              n725 = property on="Theta Go?" class="Bool (strict)"("Value"=FALSE ("Theta Go?")) -> ()  [unwired: 2 in, 2 out]
                              n726 = property on="X Go?" class="Bool (strict)"("Value"=FALSE ("X Go?")) -> ()  [unwired: 2 in, 2 out]
                              n727 = property on="Set?" class="Bool (strict)"("Value"=FALSE ("Set?")) -> ()  [unwired: 2 in, 2 out]
                              n728 = property on="X Go" class="LVObjRef (strict)"() -> ("Value"=w359:refnum<vi>)  [unwired: 2 in, 2 out]
                              n729 = property on="Z Go" class="LVObjRef (strict)"() -> ("Value"=w360:refnum<vi>)  [unwired: 2 in, 2 out]
                              n730 = property on="Theta Go" class="LVObjRef (strict)"() -> ("Value"=w361:refnum<vi>)  [unwired: 2 in, 2 out]
                              n731 = property on="Y Go" class="LVObjRef (strict)"() -> ("Value"=w358:refnum<vi>)  [unwired: 2 in, 2 out]
                              n732 = property class="Bool (strict)"(reference=w363, "Value"=FALSE) -> ()  [unwired: 1 in, 2 out]
                              n733 = property class="Bool (strict)"(reference=w359, "Value"=FALSE) -> ()  [unwired: 1 in, 2 out]
                              n734 = property class="Bool (strict)"(reference=w360, "Value"=FALSE) -> ()  [unwired: 1 in, 2 out]
                              n735 = property class="Bool (strict)"(reference=w358, "Value"=FALSE) -> ()  [unwired: 1 in, 2 out]
                              n736 = property class="Bool (strict)"(reference=w361, "Value"=FALSE) -> ()  [unwired: 1 in, 2 out]
                            }
                          }
                        }
                      }
                      n737 = case shown="No Error" w84 {
                        tunnel: w70 -> [w183 _]
                        frame No Error {
                          # "If there was no error when the motor loop began, add the error (possibly Null) to the global <Motor Error> variable.  Note:  By not checking to see if there was already an error, then this loop may continuously add errors, thus prohibiting the user from performing a clear error operation."
                          n738 = property on="Error" class="LVObjRef (strict)"() -> ("Value"=w184:refnum<vi>)  [unwired: 2 in, 2 out]
                          n739 = property class="Clust (strict)"(reference=w184, "Value"=w183) -> ()  [unwired: 1 in, 2 out]
                        }
                        frame Error {
                        }
                      }
                      "Loop i" <- w182
                    }
                  }
                }
                n740 = property on="Motors Online" class="Bool (strict)"("Value"=TRUE ("Motors Online")) -> ()  [unwired: 2 in, 2 out]
                n741 = property on="Motors Status" class="Str"("Value"="Running" ("Motors Status")) -> ()  [unwired: 2 in, 2 out]
                n742 = property on="Error" class="LVObjRef (strict)"() -> ("Value"=w50:refnum<vi>)  [unwired: 2 in, 2 out]
                n743 = property class="Clust (strict)"(reference=w50) -> (reference out=w46:refnum<vi>, "Value"=w49:errorcluster)  [unwired: 1 in, 1 out]
                n744 = call "Motors Close.vi"("error in"=w49, "VISA in"=w47) -> ("error out"=w48:errorcluster)  [unwired: 1 in]
                n745 = property class="Clust (strict)"(reference=w46, "Value"=w48) -> ()  [unwired: 1 in, 2 out]
              }
              frame Error {
                w1401 = T2 0 items=["no dialog", "OK message", "continue or stop message", "OK message + warnings", "continue/stop + warnings"] ("type of dialog (OK msg:1)")
                n746 = call <vilib>:"Simple Error Handler.vi"("type of dialog (OK msg:1)"=w1401, "error in (no error)"=w1402) -> ("error out"=w1399:errorcluster)  [unwired: 3 in, 4 out]
                n747 = property on="Motors Online" class="Bool (strict)"("Value"=FALSE ("Motors Online")) -> ()  [unwired: 2 in, 2 out]
                n748 = property class="Clust (strict)"(reference="Error", "Value"=w1399) -> ()  [unwired: 1 in, 2 out]
                n749 = Wait (ms)(milliseconds to wait=u32 1000) -> ()  [unwired: 1 out]
                n750 = property on="Motors Status" class="Str"("Value"="Motors Not Responding" ("Motors Status")) -> ()  [unwired: 2 in, 2 out]
                n751 = property on="Update Params" class="Bool (strict)"("Value"=FALSE ("Update Params")) -> ()  [unwired: 2 in, 2 out]
              }
            }
            n752 = property on="Motors Status" class="Str"("Value"="Opening Communications" ("Motors Status")) -> ()  [unwired: 2 in, 2 out]
            "Update Params" <- TRUE ("Update Params")
          }
        }
      }
    }
  }
